vi "Process.vi"(0 "reference in":refnum<class "HPS-17000-PowerModule.lvclass">, 5 "error in":errorcluster) -> (14 "reference out":refnum<class "HPS-17000-PowerModule.lvclass">, 19 "error out":errorcluster)   [LabVIEW 2023, in "HPS-17000-PowerModule.lvlib" / "HPS-17000-PowerModule.lvclass"]
uses:
  HPS-17000-PowerModule.lvclass
  HPS-17000-PowerModule.lvclass/HPS-17000-PowerModule.ctl
  <vilib>/Utility/SystemLogging/NI_SystemLogging.lvlib
  <instrlib>/HPS-17000/Client Facing Datatypes/Setpoint Stream Status Data.ctl
  <instrlib>/HPS-17000/HPS-17000.lvclass
  <instrlib>/HPS-17000/Client Facing Datatypes/Network Sync Event Data.ctl
  <instrlib>/HPS-17000/Client Facing Datatypes/Faults Event Data.ctl
  <instrlib>/HPS-17000/Client Facing Datatypes/Heartbeat Event Data.ctl
  <instrlib>/HPS-17000/Client Facing Datatypes/Multi-Cycler Events.ctl
  SSH_class/SSH.lvclass
  private/Get XC Report.vi
  private/Search HPS Network.vi
  <vilib>/HPS-17000/nibatterycycler_grpc_Setpoint.ctl
  <vilib>/HPS-17000/NI_BC_client.lvlib
  <instrlib>/HPS-17000/Client Facing Datatypes/DeviceProperties.ctl
  builds/PowerModuleInterface/PowerModuleInterface.lvlibp/Classes/PowerModule_interface/Slew Rates.ctl
  builds/PowerModuleInterface/PowerModuleInterface.lvlibp/Classes/PowerModule_interface/PowerModuleInterface.lvclass
  <instrlib>/HPS-17000/Internal/Identify Multi.vi
  <instrlib>/HPS-17000/Internal/Get Status Multi.vi
  <instrlib>/HPS-17000/Internal/Start Measurement Stream Multi.vi
  <instrlib>/HPS-17000/Internal/Start Setpoint Stream Multi.vi
  <instrlib>/HPS-17000/Internal/Stream Setpoints Multi.vi
  <instrlib>/HPS-17000/Internal/Stop Setpoint Stream Multi.vi
  <instrlib>/HPS-17000/Internal/Stop Measurement Stream Multi.vi
panel:
  in  "Main Tab Control":T1(tab)
  in  "TSN NIC IP Address":string caption="TSN NIC IP ADDRESS"
  in  "Controller TSN IP":string caption="CONTROLLER TSN IP"
  in  "HPS17K Search":bool
  in  "Device Search":string(tree) caption="HPS17K SEARCH"
  in  "HPS17K IP Addresses":string[](tree) caption="HPS17K NETWORK"
  in  "Add HPS17K":bool
  in  "Remove HPS17K":bool
  in  "HPS Topology":enum16{"SINGLE", "MULTI"}(ring) caption="HPS17K TOPOLOGY"
  out "Self Test Log":i32(listbox) caption="SELF TEST LOG"
  in  "Run Self Test":bool
  out "Test Server Log":i32(listbox) caption="TEST SERVER LOG"
  in  "Run Test Server":bool
  in  "Voltage Reformation":bool caption="REFORMATION"
  in  "Get Device Properties":bool
  in  "Get XC Report":bool
  out "Event Log":i32(listbox)=-1 caption="EVENT LOG"
  in  "Clear Event Log":bool
  in  "Volta Monitor":bool
  out "device properties":T2
  out "GM ID":string
  out "Measurement Stream":bool caption="MEASUREMENT STREAM"
  out "Setpoint Stream":bool caption="SETPOINT STREAM"
  out "OK":bool
  out "Heartbeat Valid":bool caption="HEARTBEAT VALID"
  in  "FC Sys Inspect":bool
  out "Fault Description":string caption="FAULT DESCRIPTION"
  in  "Update Temperatures":bool
  out "Temperatures":i32(listbox) caption="TEMPERATURES"
  out "Thermal Limits":i32(listbox) caption="THERMAL LIMITS"
  out "Hardware Limits":i32(listbox) caption="HARDWARE LIMITS"
  out "Last Command":string
  out "error info":errorcluster
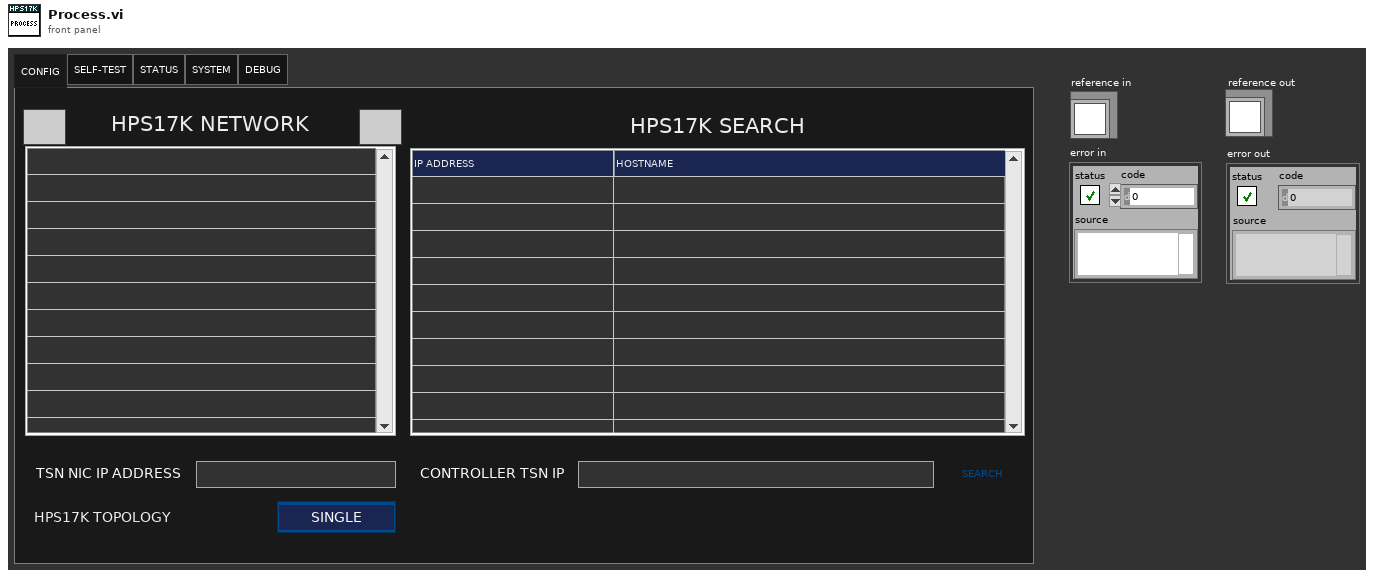
[diagram p1: front panel]
types:
  T1 = enum32{"CONFIG", "SELF-TEST", "STATUS", "SYSTEM", "DEBUG"}
  T2 = typedef "HPS-17000.lvclass/DeviceProperties.ctl" = cluster{"name":string, "model":string, "vendor":string, "serial_number":string}
  T3 = cluster{"Core":cluster{"Timeout":i32, "Events":cluster{"EventsToProcess":refnum<event-registration>, "UserEvents":refnum<event-registration>}, "EventFromProcess":refnum<user-event>, "ProcessSyncQueue":refnum<queue>, "QueueFromProcess":refnum<queue>, "Command":string, "Data":variant}, "Test Server":refnum<class "SSH.lvclass">, "Self Test":refnum<class "SSH.lvclass">, "Self Test Completed":refnum<user-event>, "Network Search Completed":refnum<user-event>, "Drag Data":cluster{"data name":string, "drag data":variant}[]}
  T4 = cluster{"data name":string, "drag data":variant}[]
  T5 = enum32{"Invalid", "Standard", "Closed", "Hidden", "Minimized", "Maximized"}
  T6 = enum8{"Enabled", "Disabled", "Disabled and Grayed Out"}
  T7 = typedef "NI_BC_client.lvlib/nibatterycycler_grpc_Setpoint.ctl" = cluster{"voltage":sgl, "current":sgl, "min_power":sgl, "max_power":sgl, "resistance":sgl}
  T8 = typedef "PowerModuleInterface.lvlibp/PowerModuleInterface.lvclass/Slew Rates.ctl" = cluster{"Current Decrease (A/sec)":dbl, "Current Increase (A/sec)":dbl, "Voltage Decrease (V/sec)":dbl, "Voltage Increase (V/sec)":dbl, "Resistance Decrease (Ohm/sec)":dbl, "Resistance Increase (Ohm/sec)":dbl}
  T9 = cluster{"EventsToProcess":refnum<event-registration>, "UserEvents":refnum<event-registration>}
  T10 = typedef "HPS-17000-PowerModule.lvlib/HPS-17000-PowerModule.lvclass/ObjectAttributes.ctl" = cluster{"JSON Config Path":path, "Configuration":T11, "GM ID":string, "HPS17000 Refs":refnum<class "HPS-17000.lvclass">[], "connected":bool, "reserved":bool, "events":T13, "nibatterycycler_grpc_Setpoint":T7, "last timestamp":i64, "mode":T14, "range":T15, "measurement array":T16[], "measurement stream":bool, "setpoint stream":bool}
  T11 = typedef "HPS-17000-PowerModule.lvlib/HPS-17000-PowerModule.lvclass/Configuration.ctl" = cluster{"TSN NIC IP Address":string, "HPS17000 IP Addresses":string[], "HPS Topology":enum16{"SINGLE", "MULTI"}, "Setpoint Stream Config":T12, "Measurement Array Size":i32, "Read Timeout (ms)":i32}
  T12 = typedef "Cycler.lvclass/Setpoint Stream Basic Config.ctl" = cluster{"local address":string, "receiver port":u16}
  T13 = typedef "HPS-17000.lvclass/Multi-Cycler Events.ctl" = cluster{"heartbeats events":refnum<user-event>[], "faults events":refnum<user-event>[], "network sync event":refnum<user-event>[], "setpoint status event":refnum<user-event>[]}
  T14 = typedef "HPS-17000-PowerModule.lvlib/HPS-17000-PowerModule.lvclass/Mode.ctl" = u16
  T15 = typedef "PowerModuleInterface.lvlibp/PowerModuleInterface.lvclass/Range.ctl" = cluster{"Current Max (A)":dbl, "Current Min (A)":dbl, "Voltage Max (V)":dbl, "Voltage Min (V)":dbl}
  T16 = typedef "PowerModuleInterface.lvlibp/PowerModuleInterface.lvclass/Measurements.ctl" = cluster{"measured voltage (V)":dbl, "measured current (A)":dbl, "setpoint voltage (V)":dbl, "setpoint current (A)":dbl, "timestamp":dbl}
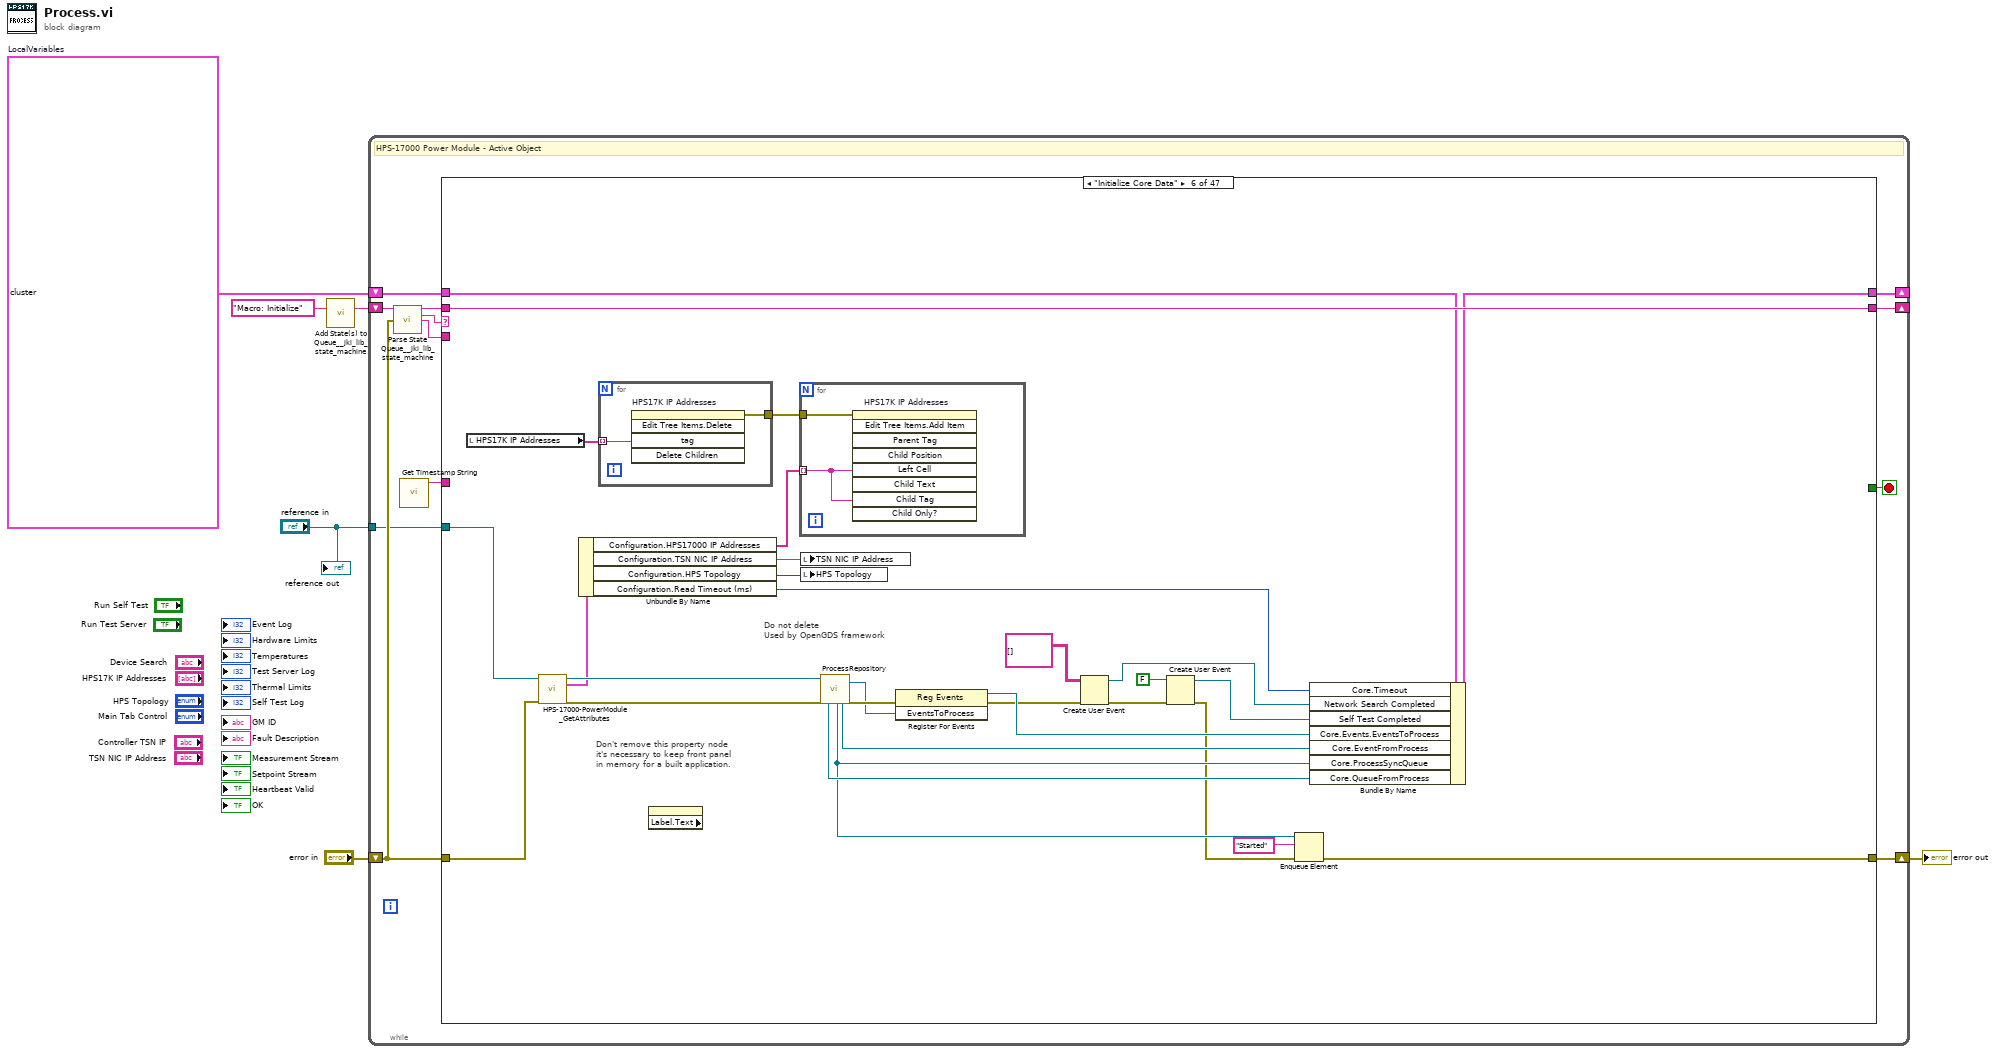
[diagram p0: block diagram]
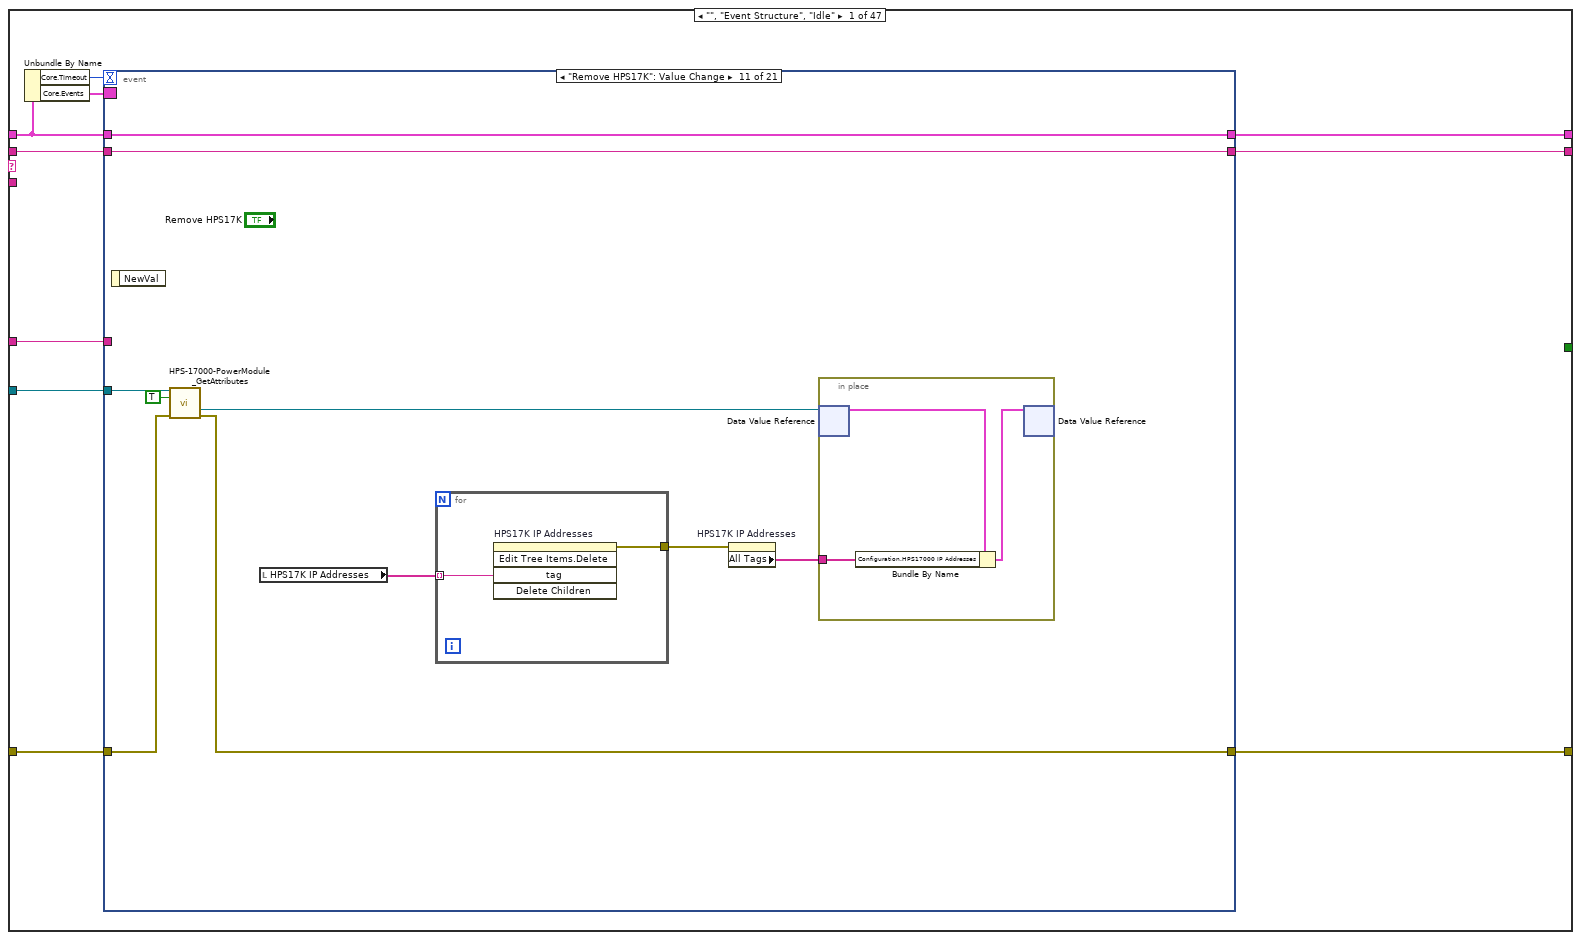
[diagram p2: hidden frame]
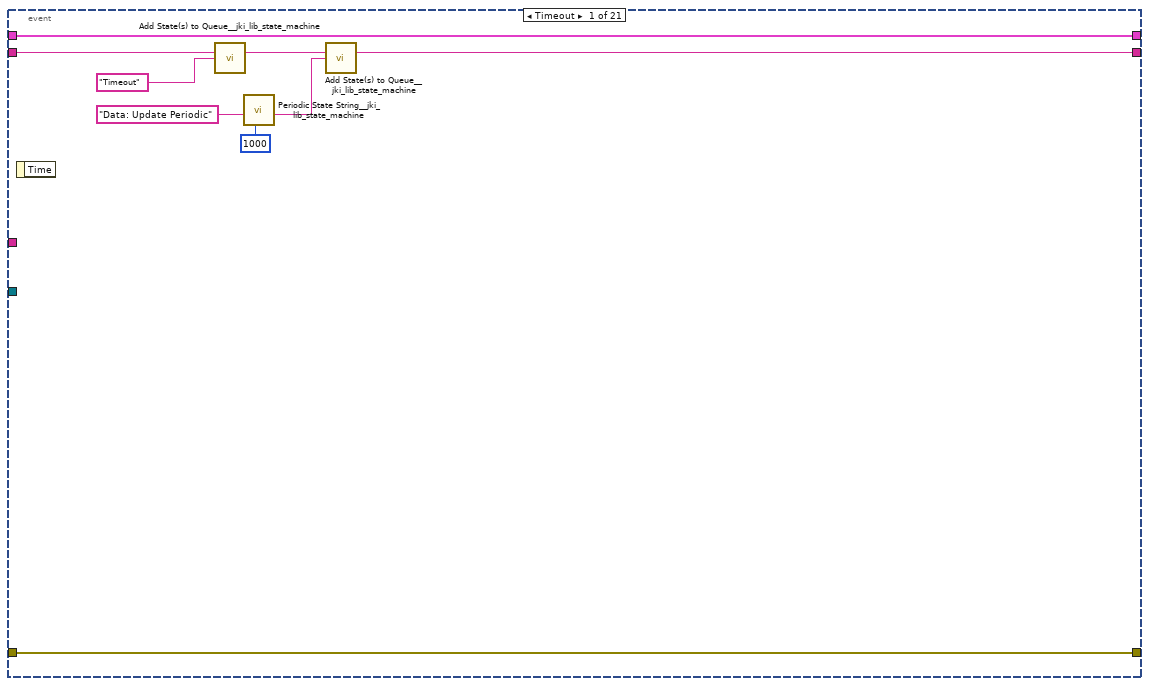
[diagram p3: hidden frame]
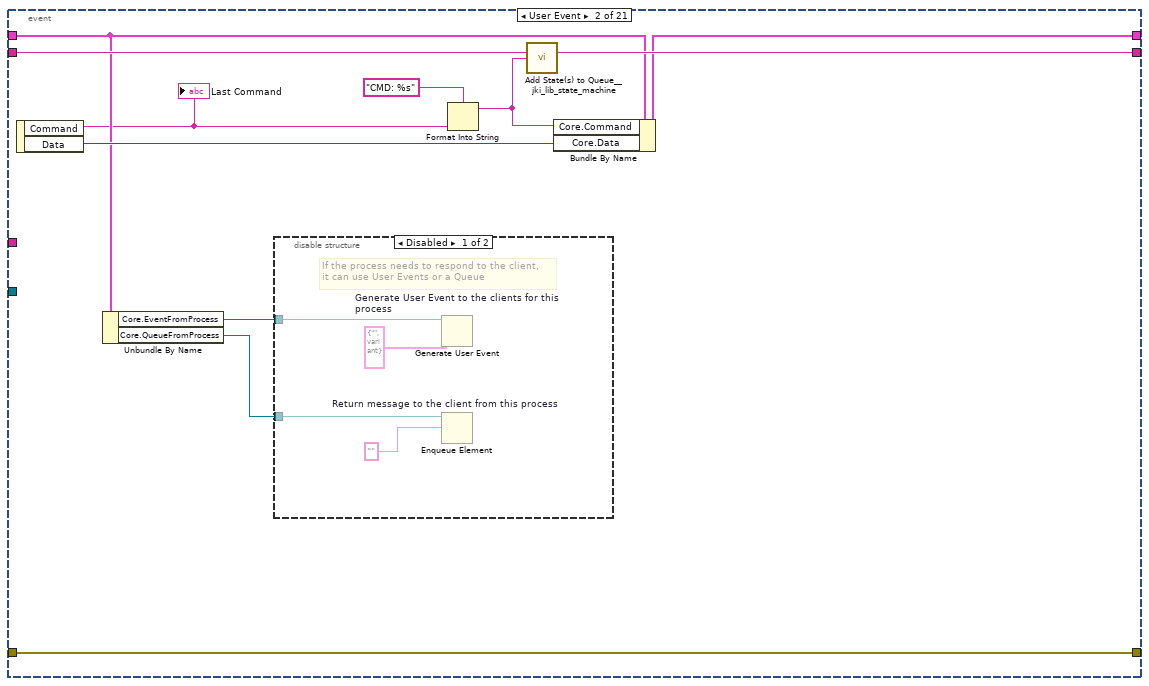
[diagram p4: hidden frame]
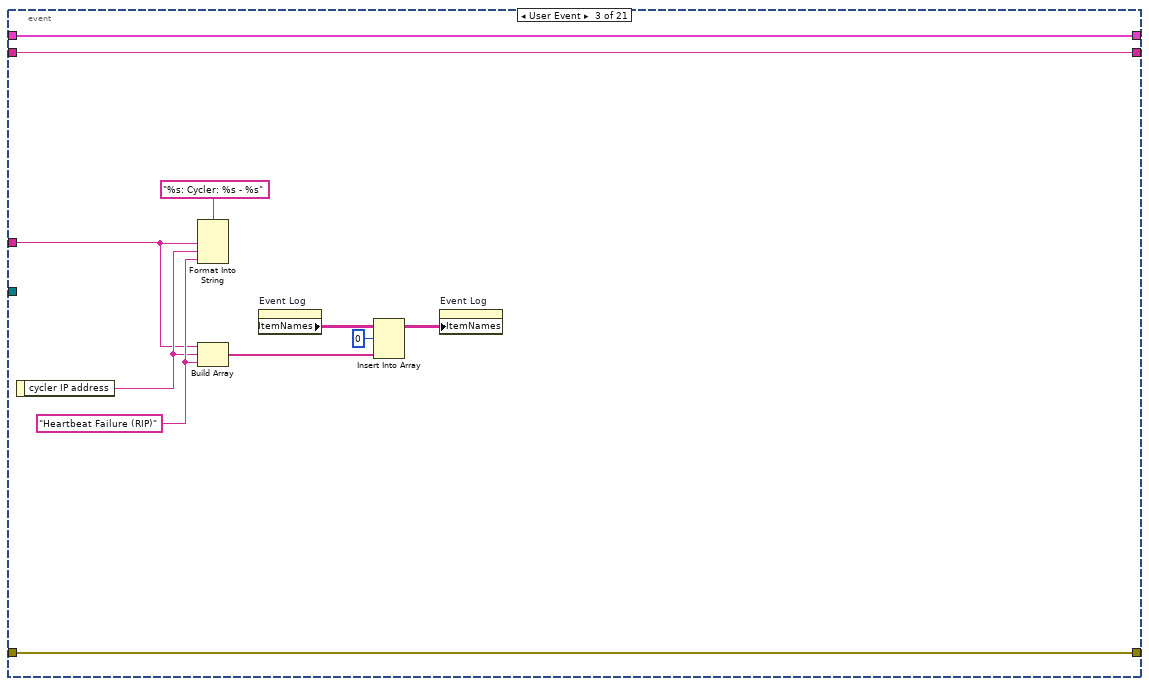
[diagram p6: hidden frame]
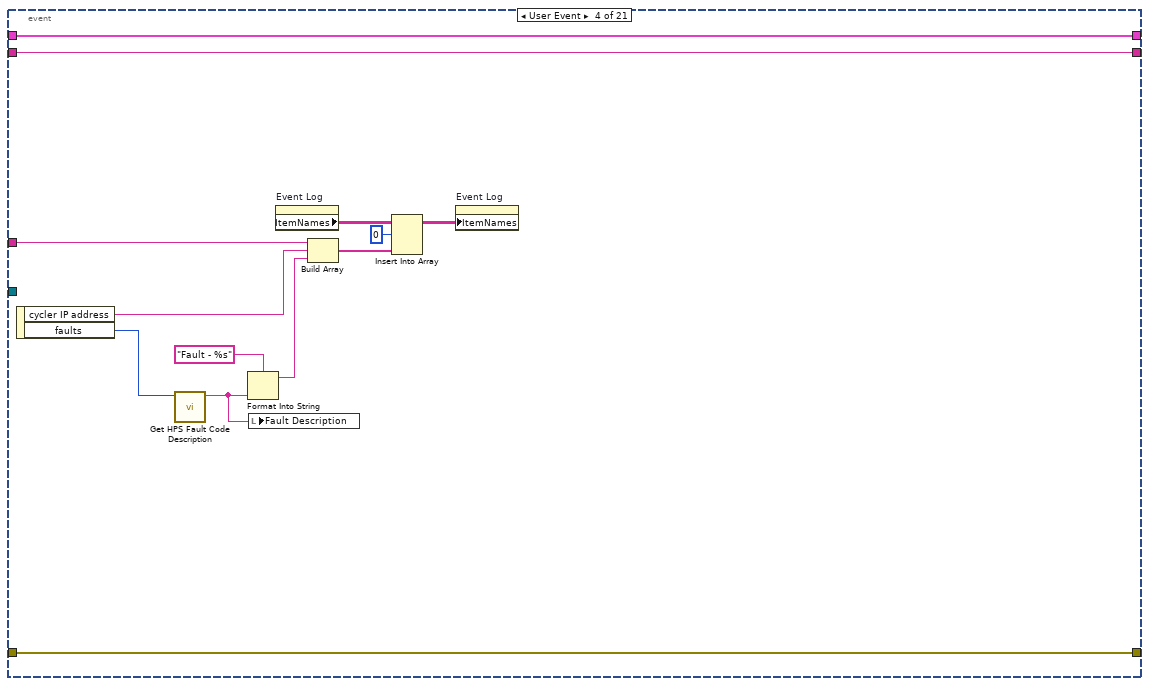
[diagram p7: hidden frame]
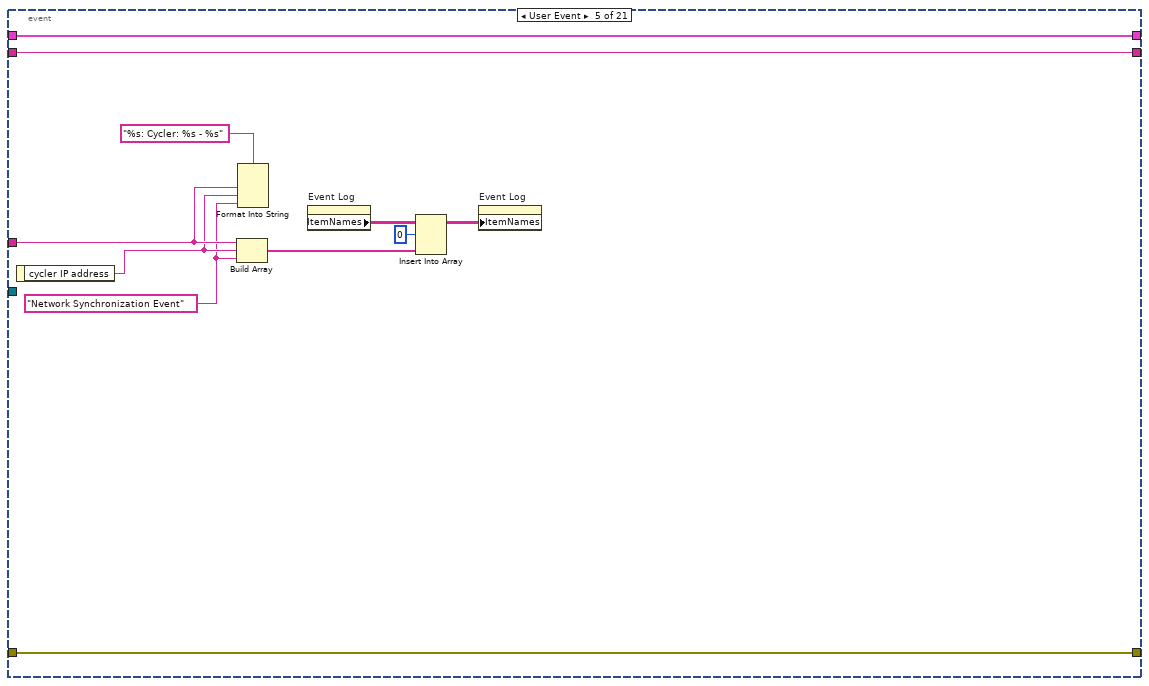
[diagram p8: hidden frame]
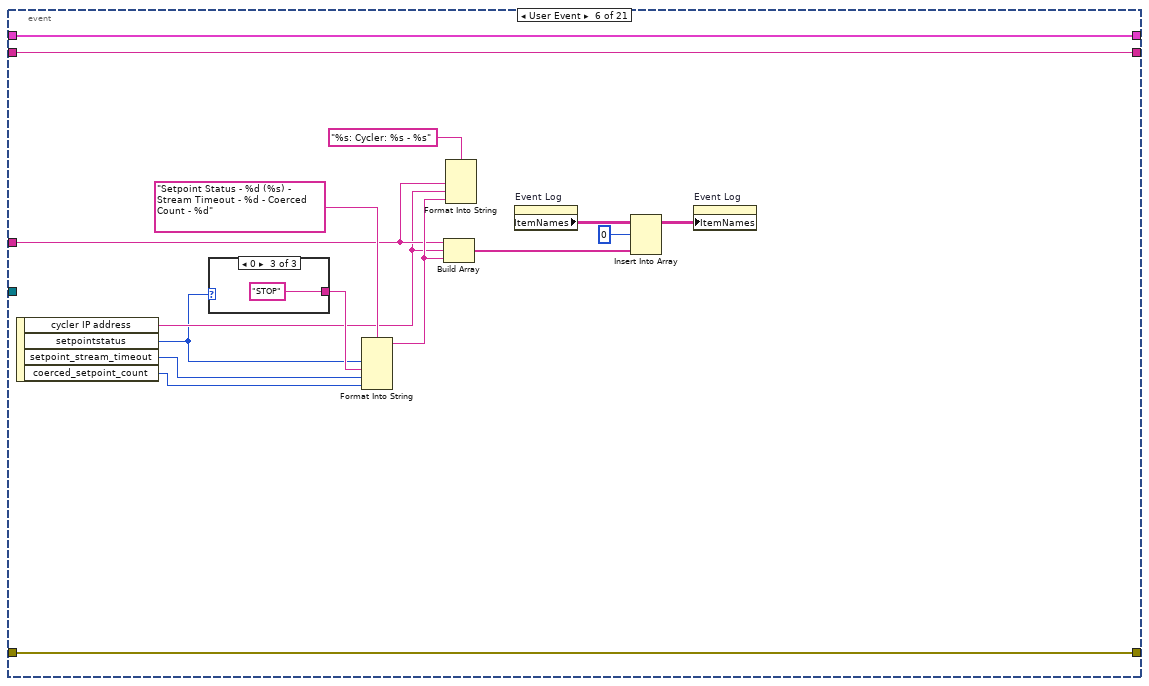
[diagram p9: hidden frame]
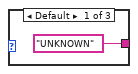
[diagram p10: hidden frame]
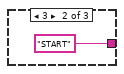
[diagram p11: hidden frame]
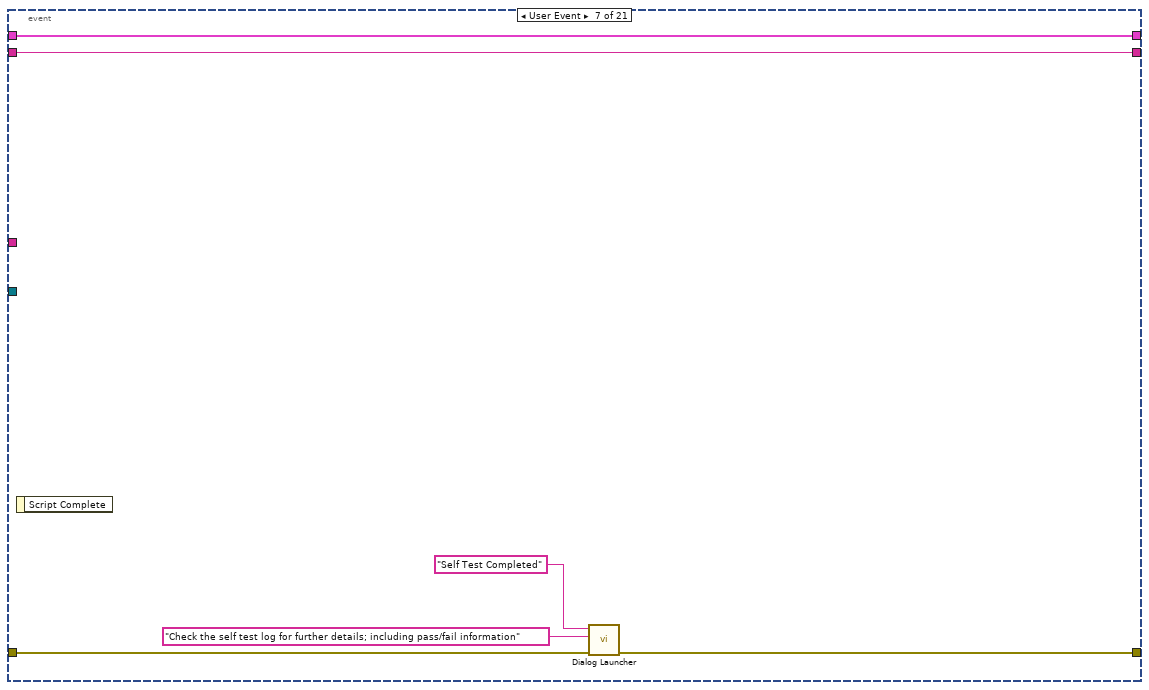
[diagram p12: hidden frame]
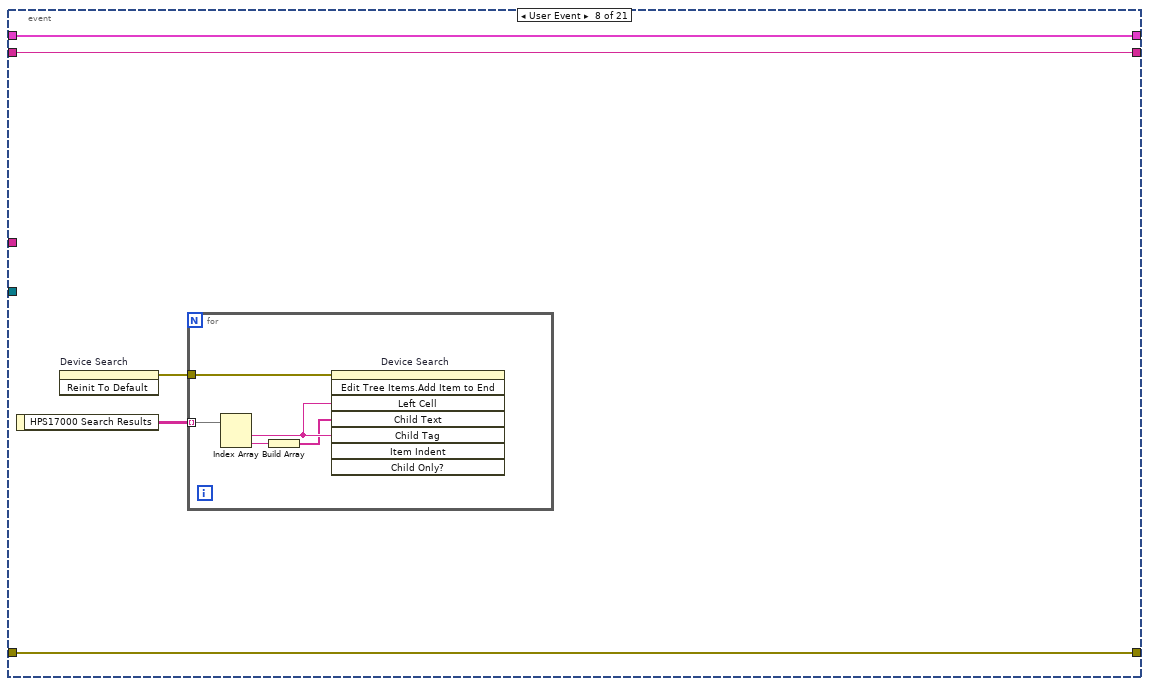
[diagram p13: hidden frame]
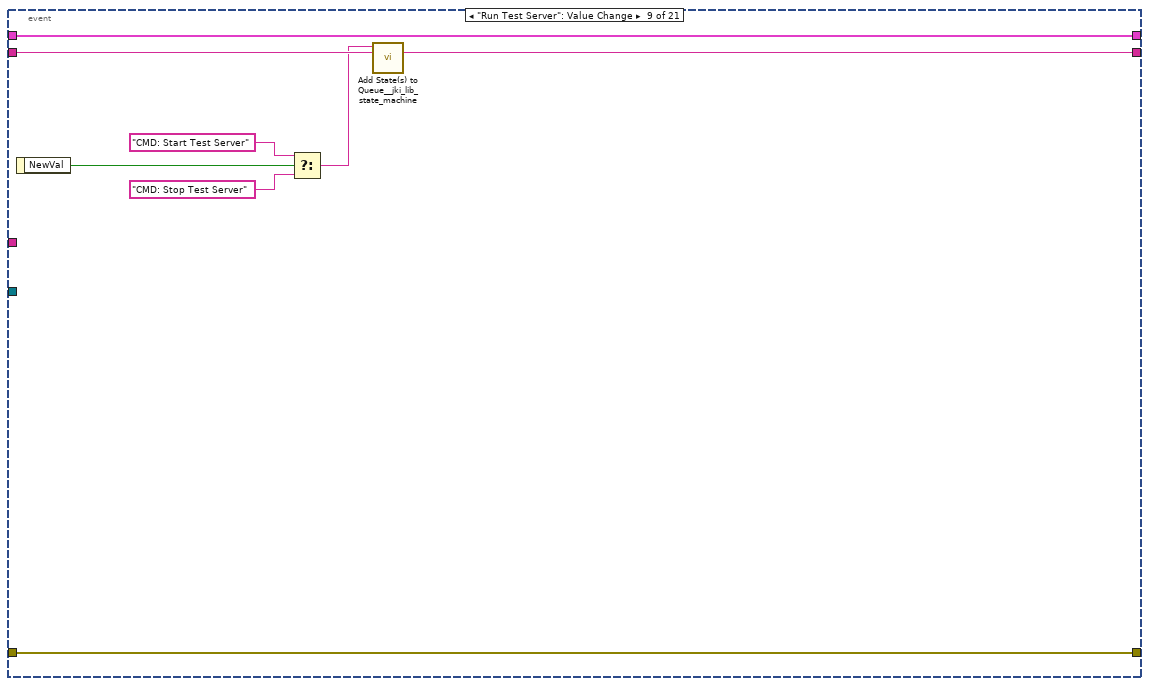
[diagram p14: hidden frame]
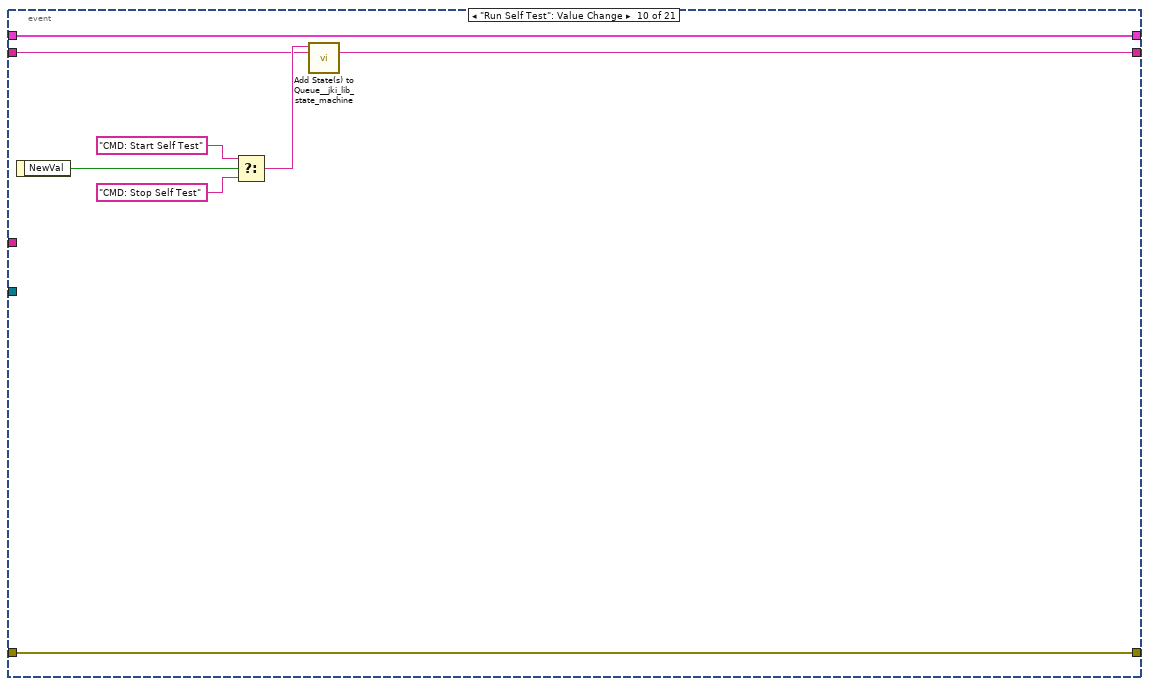
[diagram p15: hidden frame]
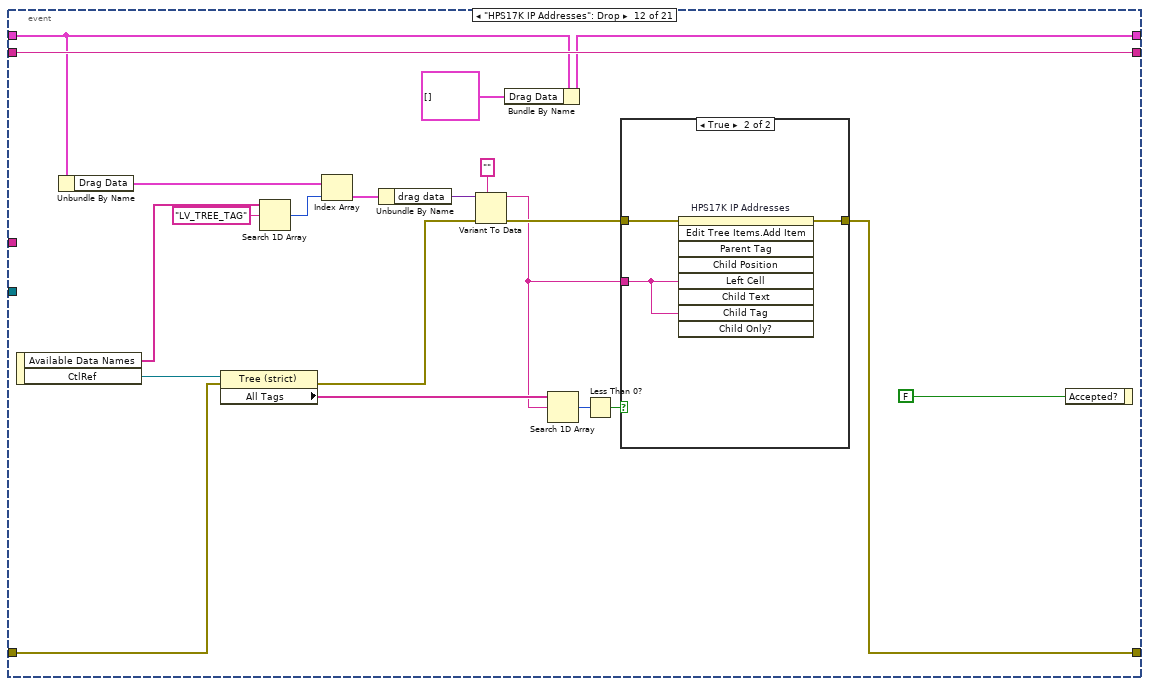
[diagram p16: hidden frame]
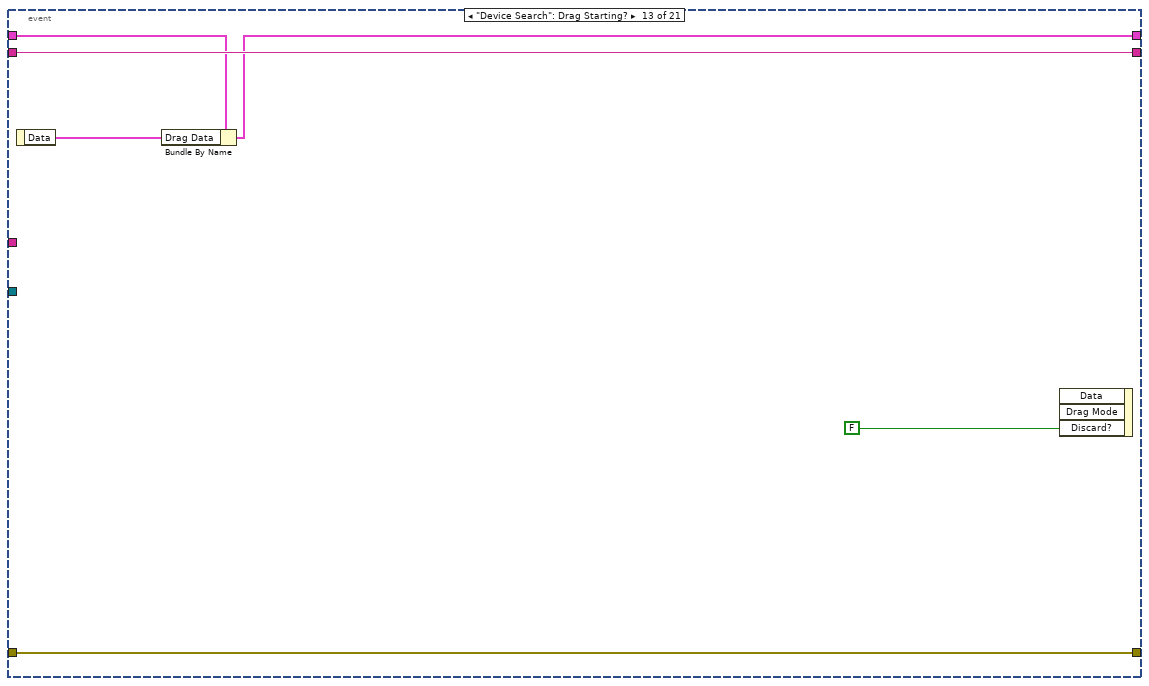
[diagram p18: hidden frame]
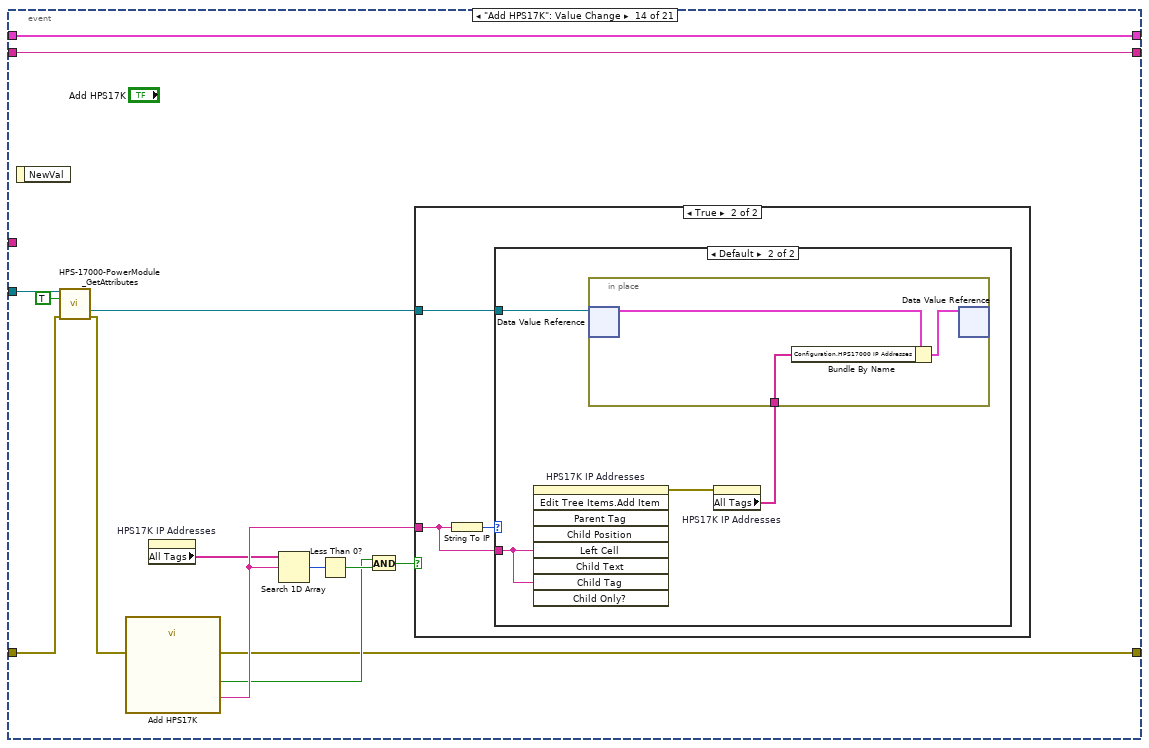
[diagram p19: hidden frame]
diagram:
  w6 = T3 {"Core"={"Timeout"=-1, "Events"={"EventsToProcess"=refnum, "UserEvents"=refnum}, "EventFromProcess"=refnum, "ProcessSyncQueue"=refnum, "QueueFromProcess"=refnum, "Command"="", "Data"=variant}, "Test Server"=refnum, "Self Test"=refnum, "Self Test Completed"=refnum, "Network Search Completed"=refnum, "Drag Data"=[]}  # LocalVariables
  n1 = call <vilib>:"Add State(s) to Queue__jki_lib_state_machine.vi"("State(s) in (\"\")"="Macro: Initialize" ("States Out")) -> ("States Out"=w2:string)  [unwired: 14 in]
  n2 = while {
    shift-right: [w17] -> w5
    shift-left: "error in" -> [w18]
    shift-right: [w10] -> _
    shift-left: w2 -> [w13]
    shift-right: [w16] -> _
    shift-left: w6 -> [w15]
    tunnel: "reference in" -> [w8]
    stop <- w9 stop-if-true
    # "HPS-17000 Power Module - Active Object"
    n3 = call <vilib>:"Parse State Queue__jki_lib_state_machine.vi"("State Queue"=w13, "Error In (no error)"=w18) -> ("Remaining States"=w12:string, "Current State"=w14:string, "Arguments"=w11:string)  [unwired: 11 in]
    n4 = call "Get Timestamp String.vi"() -> ("date/time string"=w7:string)  [unwired: 11 in]
    n5 = case shown="\"Initialize Core Data\"" w14 {
      selector: w14 -> [_ _ w291 _ _ _ _ _ _ _ _ _ _ _ _ _ _ _ _ _ _ _ _ _ _ _ _ _ _ _ _ _ _ _ _ _ _ _ _ _ _ _ _ _ _ _ _]
      tunnel: w18 -> [w24 w290 w293 w313 w382 w399 w418 w442 w455 w456 w486 _ w492 w506 w510 w514 w519 w524 w527 w534 w539 w554 w581 w604 w634 w661 w677 w701 w729 w745 w758 w766 w777 w795 w814 w822 w838 w841 w846 w851 w856 w861 w866 w871 w876 w881 w886]
      tunnel: [w22 w290 w292 w308 errorcluster {"status"=FALSE, "code"=0, "source"=""} ("error constant") w413 w425 w438 w455 w456 w486 w487 w491 w506 w510 w514 w519 w524 w527 w534 w546 w553 w580 w601 w631 w658 w674 w698 w725 w741 w757 w765 w776 w782 w817 w825 w838 w841 w846 w851 w856 w861 w866 w871 w876 w881 w886] -> w17
      tunnel: [w28 w289 w300 w302 w384 w411 w426 w444 w454 w458 w478 w488 w495 w505 w509 w513 w518 w523 w526 w533 w544 w548 w579 w607 w637 w664 w680 w704 w724 w740 w763 w771 w779 w794 w819 w823 w837 w840 w845 w850 w855 w860 w865 w870 w875 w880 w885] -> w16
      tunnel: w15 -> [w25 w289 w300 w302 w384 w410 w426 w444 w454 w458 w478 w488 w495 w505 w509 w513 w518 w523 w526 w533 w545 w549 w578 w607 w637 w664 w680 w704 w723 w739 w763 w771 w779 w794 w819 w823 w837 w840 w845 w850 w855 w860 w865 w870 w875 w880 w885]
      tunnel: w12 -> [w27 w288 w299 w301 w383 w412 w429 w445 w453 w459 w485 w490 w494 w504 w508 w512 w517 w522 _ w532 w547 w555 w582 w606 w636 w663 w679 w703 w730 w746 w762 w770 w778 w797 w820 w824 w836 w839 w844 w849 w854 w859 w864 w869 w874 w879 w884]
      tunnel: w11 -> [_ _ _ _ _ _ _ _ _ w457 _ _ w493 _ _ _ _ _ _ w529 _ _ _ _ _ _ _ _ _ _ _ _ _ _ _ _ _ _ _ _ _ _ _ _ _ _ _]
      tunnel: [w26 w288 w299 w301 w383 w412 w429 w445 w453 w459 w485 w490 w494 w504 w508 w512 w516 w521 "Macro: Exit" ("State(s) at Back (\"\")") w531 w547 w555 w582 w606 w636 w663 w679 w703 w730 w746 w762 w770 w778 w797 w820 w824 w836 w839 w842 w848 w853 w858 w863 w868 w873 w878 w883] -> w10
      tunnel: [_ _ _ _ _ _ TRUE _ _ _ _ _ _ _ _ _ _ _ _ _ _ _ _ _ _ _ _ _ _ _ _ _ _ _ _ _ _ _ _ _ _ _ _ _ _ _ _] -> w9
      tunnel: w8 -> [w19 _ _ w314 _ w402 _ w443 _ _ _ _ _ _ _ _ _ _ _ _ w540 _ _ w605 w635 w662 w678 w702 _ _ _ _ _ _ _ w827 _ _ _ _ _ _ _ _ _ _ _]
      tunnel: w7 -> [w20 _ _ _ _ _ _ _ _ _ _ _ _ _ _ _ _ _ _ _ _ _ _ _ _ _ _ _ _ _ _ _ _ _ _ _ _ _ _ _ _ _ _ _ _ _ _]
      frame "", "Event Structure", "Idle" {
        n6 = Unbundle By Name(w25) -> ("Core.Timeout"=w23:i32, "Core.Events"=w21:T9)
        n7 = event shown="[10] \"Remove HPS17K\": Value Change" {
          selector: w21 -> [_ _ _ _ _ _ _ _ _ _ _ _ _ _ _ _ _ _ _ _ _]
          dyn-events: _ -> [_ _ _ _ _ _ _ _ _ _ _ _ _ _ _ _ _ _ _ _ _]
          timeout: w23 -> [_ _ _ _ _ _ _ _ _ _ _ _ _ _ _ _ _ _ _ _ _]
          tunnel: w25 -> [w37 w41 w63 w76 w87 w103 w112 w117 w130 w138 w148 w161 w181 w198 w218 w228 w238 w245 w278 w282 w287]
          tunnel: [w37 w46 w63 w76 w87 w103 w112 w117 w130 w138 w148 w160 w180 w198 w218 w228 w238 w245 w278 w282 w287] -> w28
          tunnel: [w29 w48 w62 w75 w86 w102 w111 w116 w127 w131 w147 w174 w184 w197 w217 w227 w237 w247 w274 w281 w283] -> w26
          tunnel: w27 -> [w36 w47 w62 w75 w86 w102 w111 w116 w128 w132 w147 w174 w184 w197 w217 w227 w237 w247 w276 w281 w285]
          tunnel: [w34 w42 w61 w74 w85 w101 w107 w115 w129 w137 w143 w154 w183 w191 w215 w226 w235 w246 w277 w280 w286] -> w22
          tunnel: w24 -> [w34 w42 w61 w74 w85 w101 w110 w115 w129 w137 w144 w167 w183 w188 w216 w224 w236 w241 w277 w280 w286]
          tunnel: w20 -> [_ _ w53 w66 w80 w94 _ _ _ _ _ _ _ _ _ _ _ _ _ _ _]
          tunnel: w19 -> [_ _ _ _ _ _ _ _ _ _ w146 _ _ w189 _ w225 _ w242 _ _ _]
          event Timeout {
            n8 = event-data() -> ()  [unwired: 1 in, 1 out]
            n9 = call <vilib>:"Add State(s) to Queue__jki_lib_state_machine.vi"("State(s) in (\"\")"=w36, "State(s) at Back (\"\")"="Timeout" ("State(s) at Back (\"\")")) -> ("States Out"=w32:string)  [unwired: 13 in]
            n10 = call <vilib>:"Periodic State String__jki_lib_state_machine.vi"("Period (ms)"=u32 1000, "State"="Data: Update Periodic") -> ("State Out"=w31:string)  [unwired: 9 in]
            n11 = call <vilib>:"Add State(s) to Queue__jki_lib_state_machine.vi"("State(s) in (\"\")"=w32, "State(s) at Back (\"\")"=w31) -> ("States Out"=w29:string)  [unwired: 13 in]
          }
          event User Event {
            n12 = event-data() -> ("Command"=w39:string, "Data"=w45:variant)  [unwired: 1 in]
            "Last Command" <- w39
            n13 = Unbundle By Name(w41) -> ("Core.EventFromProcess"=w44:refnum<user-event>, "Core.QueueFromProcess"=w43:refnum<queue>)
            n14 = disable-structure shown="Disabled" {
              disable-tunnel: w44 -> [w52 _]
              disable-tunnel: w43 -> [w51 _]
              frame Disabled {
                # "If the process needs to respond to the client,\nit can use User Events or a Queue"
                n15 = Generate User Event "Generate User Event to the clients for this process"(user event=w52, event data cluster=cluster{"Command":string, "Data":variant} {"Command"="", "Data"=variant} ("event data")) -> ()  [unwired: 2 in, 2 out]
                n16 = Enqueue Element "Return message to the client from this process"(queue=w51, element="") -> ()  [unwired: 2 in, 3 out]
              }
              frame Enabled {
              }
            }
            n17 = Format Into String(format string="CMD: %s", w39) -> (resulting string=w38:string)  [unwired: 2 in, 1 out]
            n18 = call <vilib>:"Add State(s) to Queue__jki_lib_state_machine.vi"("State(s) in (\"\")"=w47, "State(s) at Back (\"\")"=w38) -> ("States Out"=w48:string)  [unwired: 13 in]
            n19 = Bundle By Name(cluster=w41, "Core.Command"=w38, "Core.Data"=w45) -> (w46:T3)
          }
          event User Event {
            w56 = "Heartbeat Failure (RIP)" ("format string")
            n20 = event-data() -> ("cycler IP address"=w55:string)  [unwired: 1 in]
            n21 = Format Into String(format string="%s: Cycler: %s - %s", w53, w55, w56) -> ()  [unwired: 2 in, 2 out]
            n22 = Build Array(w53, w55, w56) -> (w59:string[])
            n23 = property on="Event Log" class="MCListbox (strict)"() -> ("ItemNames"=w60:string[][])  [unwired: 2 in, 2 out]
            n24 = Insert Into Array(array=w60, index (row)=0, new element=w59) -> (w54:string[][])  [unwired: 1 in]
            n25 = property on="Event Log" class="MCListbox (strict)"("ItemNames"=w54) -> ()  [unwired: 2 in, 2 out]
          }
          event User Event {
            n26 = event-data() -> ("cycler IP address"=w67:string, "faults"=w68:u64)  [unwired: 1 in]
            n27 = call "Get HPS Fault Code Description.vi"("fault code"=w68) -> ("fault description"=w69:string)  [unwired: 10 in]
            n28 = Format Into String(format string="Fault - %s", w69) -> (resulting string=w72:string)  [unwired: 2 in, 1 out]
            n29 = local write "Fault Description"(w69) -> ()
            n30 = property on="Event Log" class="MCListbox (strict)"() -> ("ItemNames"=w65:string[][])  [unwired: 2 in, 2 out]
            n31 = Build Array(w66, w67, w72) -> (w70:string[])
            n32 = Insert Into Array(array=w65, index (row)=0, new element=w70) -> (w64:string[][])  [unwired: 1 in]
            n33 = property on="Event Log" class="MCListbox (strict)"("ItemNames"=w64) -> ()  [unwired: 2 in, 2 out]
          }
          event User Event {
            w78 = "Network Synchronization Event" ("format string")
            n34 = event-data() -> ("cycler IP address"=w79:string)  [unwired: 1 in]
            n35 = Build Array(w80, w79, w78) -> (w77:string[])
            n36 = Format Into String(format string="%s: Cycler: %s - %s", w80, w79, w78) -> ()  [unwired: 2 in, 2 out]
            n37 = property on="Event Log" class="MCListbox (strict)"() -> ("ItemNames"=w84:string[][])  [unwired: 2 in, 2 out]
            n38 = Insert Into Array(array=w84, index (row)=0, new element=w77) -> (w83:string[][])  [unwired: 1 in]
            n39 = property on="Event Log" class="MCListbox (strict)"("ItemNames"=w83) -> ()  [unwired: 2 in, 2 out]
          }
          event User Event {
            n40 = event-data() -> ("cycler IP address"=w93:string, "setpointstatus"=w92:i32, "setpoint_stream_timeout"=w91:u32, "coerced_setpoint_count"=w90:u32)  [unwired: 1 in]
            n41 = case shown="0" w92 {
              tunnel: ["UNKNOWN" ("input 2") "START" ("input 2") "STOP" ("input 2")] -> w95
              frame Default {
              }
              frame 3 {
              }
              frame 0 {
              }
            }
            n42 = Format Into String(format string="Setpoint Status - %d (%s) - Stream Timeout - %d - Coerced Count - %d", w92, w95, w91, w90) -> (resulting string=w96:string)  [unwired: 2 in, 1 out]
            n43 = Build Array(w94, w93, w96) -> (w100:string[])
            n44 = Format Into String(format string="%s: Cycler: %s - %s", w94, w93, w96) -> ()  [unwired: 2 in, 2 out]
            n45 = property on="Event Log" class="MCListbox (strict)"() -> ("ItemNames"=w89:string[][])  [unwired: 2 in, 2 out]
            n46 = Insert Into Array(array=w89, index (row)=0, new element=w100) -> (w88:string[][])  [unwired: 1 in]
            n47 = property on="Event Log" class="MCListbox (strict)"("ItemNames"=w88) -> ()  [unwired: 2 in, 2 out]
          }
          event User Event {
            n48 = event-data() -> ()  [unwired: 1 in, 1 out]
            n49 = call "Dialog Launcher.vi"("error in (no error)"=w110, "Message"="Check the self test log for further details; including pass/fail information", "Title"="Self Test Completed") -> ("error out"=w107:errorcluster)  [unwired: 8 in]
          }
          event User Event {
            n50 = event-data() -> ("HPS17000 Search Results"=w113:string[][])  [unwired: 1 in]
            n51 = invoke on="Device Search" class="Tree (strict)" method="Reinit To Default"() -> (error out=w114:errorcluster)  [unwired: 3 in, 2 out]
            n52 = for {
              tunnel: w114 -> [w122]
              tunnel: w113 -> [w121] mode=indexing
              n53 = Index Array(array=w121) -> (element #1=w120:string, element #2=w119:string)  [unwired: 2 in]
              n54 = Build Array(w119) -> (w118:string[])
              n55 = invoke on="Device Search" class="Tree (strict)" method="Edit Tree Items.Add Item to End"(error in=w122, "Left Cell"=w120, "Child Text"=w118, "Child Tag"=w120) -> ()  [unwired: 4 in, 8 out]
            }
          }
          event "Run Test Server": Value Change {
            n56 = event-data() -> ("NewVal"=w125:bool)  [unwired: 1 in]
            n57 = Select(t="CMD: Start Test Server" ("State(s) in Front (\"\")"), s=w125, f="CMD: Stop Test Server" ("State(s) in Front (\"\")")) -> (s? t:f=w123:string)
            n58 = call <vilib>:"Add State(s) to Queue__jki_lib_state_machine.vi"("State(s) in Front (\"\")"=w123, "State(s) in (\"\")"=w128) -> ("States Out"=w127:string)  [unwired: 13 in]
          }
          event "Run Self Test": Value Change {
            n59 = event-data() -> ("NewVal"=w134:bool)  [unwired: 1 in]
            n60 = Select(t="CMD: Start Self Test" ("State(s) in Front (\"\")"), s=w134, f="CMD: Stop Self Test" ("State(s) in Front (\"\")")) -> (s? t:f=w133:string)
            n61 = call <vilib>:"Add State(s) to Queue__jki_lib_state_machine.vi"("State(s) in Front (\"\")"=w133, "State(s) in (\"\")"=w132) -> ("States Out"=w131:string)  [unwired: 13 in]
          }
          event "Remove HPS17K": Value Change {
            n62 = event-data() -> ()  [unwired: 1 in, 1 out]
            n63 = call "HPS-17000-PowerModule_GetAttributes.vi"("reference in"=w146, "OnlyGetDvrReference(False)"=TRUE, "Error In"=w144) -> ("DataRef"=w140:refnum<data-value>, "Error Out"=w143:errorcluster)  [unwired: 9 in, 2 out]
            n64 = local read "HPS17K IP Addresses"() -> (w142:string[])
            n65 = for {
              tunnel: w142 -> [w153] mode=indexing
              tunnel: [w152] -> w141
              n66 = invoke on="HPS17K IP Addresses" class="Tree (strict)" method="Edit Tree Items.Delete"("tag"=w153) -> (error out=w152:errorcluster)  [unwired: 4 in, 4 out]
            }
            n67 = property on="HPS17K IP Addresses" class="Tree (strict)"(error in=w141) -> ("All Tags"=w139:string[])  [unwired: 1 in, 2 out]
            n68 = in-place {
              in-place-border: w139 -> [w149]
              n69 = in-place-dvr #1(w140) -> (w151:T10)  [unwired: 1 out]
              n70 = Bundle By Name(cluster=w151, "Configuration.HPS17000 IP Addresses"=w149) -> (w150:T10)
              n71 = in-place-dvr #1(w150) -> ()  [unwired: 2 out]
            }
          }
          event "HPS17K IP Addresses": Drop {
            n72 = event-data() -> ("Available Data Names"=w173:string[], "CtlRef"=w168:refnum<vi>)  [unwired: 1 in]
            n73 = Unbundle By Name(w161) -> ("Drag Data"=w171:T4)
            n74 = property class="Tree (strict)"(reference=w168, error in=w167) -> (error out=w166:errorcluster, "All Tags"=w163:string[])  [unwired: 1 out]
            n75 = Search 1D Array(1D array=w173, element="LV_TREE_TAG") -> (index of element=w170:i32)  [unwired: 1 in]
            n76 = Index Array(array=w171, index=w170) -> (element=w169:cluster{"data name":string, "drag data":variant})
            n77 = Unbundle By Name(w169) -> ("drag data"=w165:variant)
            n78 = Variant To Data(error in=w166, type="", Variant=w165) -> (data=w155:string, error out=w158:errorcluster)
            n79 = Bundle By Name(cluster=w161, "Drag Data"=T4 []) -> (w160:T3)
            n80 = Search 1D Array(1D array=w163, element=w155) -> (index of element=w157:i32)  [unwired: 1 in]
            n81 = Less Than 0?(x=w157) -> (x < 0?=w156:bool)
            n82 = case shown="True" w156 {
              tunnel: w158 -> [w175 w178]
              tunnel: w155 -> [_ w177]
              tunnel: [w175 w176] -> w154
              frame False {
              }
              frame True {
                n83 = invoke on="HPS17K IP Addresses" class="Tree (strict)" method="Edit Tree Items.Add Item"(error in=w178, "Left Cell"=w177, "Child Tag"=w177) -> (error out=w176:errorcluster)  [unwired: 6 in, 8 out]
              }
            }
            n84 = event-data("Accepted?"=FALSE) -> ()  [unwired: 1 in, 1 out]
          }
          event "Device Search": Drag Starting? {
            n85 = event-data() -> ("Data"=w179:T4)  [unwired: 1 in]
            n86 = Bundle By Name(cluster=w181, "Drag Data"=w179) -> (w180:T3)
            n87 = event-data("Discard?"=FALSE) -> ()  [unwired: 3 in, 1 out]
          }
          event "Add HPS17K": Value Change {
            n88 = event-data() -> ()  [unwired: 1 in, 1 out]
            n89 = call "HPS-17000-PowerModule_GetAttributes.vi"("reference in"=w189, "OnlyGetDvrReference(False)"=TRUE, "Error In"=w188) -> ("DataRef"=w185:refnum<data-value>, "Error Out"=w187:errorcluster)  [unwired: 9 in, 2 out]
            n90 = call "Add HPS17K"("error in (no error)"=w187) -> ("IP Address"=w196:string, "Add"=w193:bool, "error out"=w191:errorcluster)  [unwired: 16 in]
            n91 = property on="HPS17K IP Addresses" class="Tree (strict)"() -> ("All Tags"=w190:string[])  [unwired: 2 in, 2 out]
            n92 = Search 1D Array(1D array=w190, element=w196) -> (index of element=w195:i32)  [unwired: 1 in]
            n93 = Less Than 0?(x=w195) -> (x < 0?=w194:bool)
            n94 = And(x=w193, y=w194) -> (x .and. y?=w192:bool)
            n95 = case shown="True" w192 {
              tunnel: w196 -> [_ w200]
              tunnel: w185 -> [_ w199]
              frame False {
              }
              frame True {
                n96 = String To IP(1:w200) -> (0:w201:u32)
                n97 = case shown="Default" w201 {
                  tunnel: w200 -> [_ w205]
                  tunnel: w199 -> [_ w204]
                  frame 0, 181174352 {
                    # "0 = invalid\n\n181174352 = empty (localhost?)"
                  }
                  frame Default {
                    n98 = invoke on="HPS17K IP Addresses" class="Tree (strict)" method="Edit Tree Items.Add Item"("Left Cell"=w205, "Child Tag"=w205) -> (error out=w203:errorcluster)  [unwired: 7 in, 8 out]
                    n99 = property on="HPS17K IP Addresses" class="Tree (strict)"(error in=w203) -> ("All Tags"=w202:string[])  [unwired: 1 in, 2 out]
                    n100 = in-place {
                      in-place-border: w202 -> [w206]
                      n101 = in-place-dvr #2(w204) -> (w208:T10)  [unwired: 1 out]
                      n102 = Bundle By Name(cluster=w208, "Configuration.HPS17000 IP Addresses"=w206) -> (w207:T10)
                      n103 = in-place-dvr #2(w207) -> ()  [unwired: 2 out]
                    }
                  }
                }
              }
            }
          }
          event "Volta Monitor": Value Change {
            n104 = event-data() -> ()  [unwired: 1 in, 1 out]
            n105 = property on="HPS17K IP Addresses" class="Tree (strict)"() -> ("All Tags"=w209:string[])  [unwired: 2 in, 2 out]
            n106 = Index Array(array=w209) -> (element=w210:string)  [unwired: 1 in]
            n107 = Format Into String(format string="plink -l admin %s -batch -t \"/usr/local/natinst/bin/volta_monitor\"", w210) -> (resulting string=w213:string)  [unwired: 2 in, 1 out]
            n108 = call <vilib>:"System Exec.vi"("run minimized? (F)"=FALSE, "wait until completion? (T)"=FALSE, "error in (no error)"=w216, "command line"=w213) -> ("error out"=w215:errorcluster)  [unwired: 4 in, 3 out]
          }
          event "Get Device Properties": Value Change {
            n109 = event-data() -> ()  [unwired: 1 in, 1 out]
            n110 = call "HPS-17000-PowerModule_GetAttributes.vi"("reference in"=w225, "Error In"=w224) -> ("Data"=w222:T10, "Error Out"=w223:errorcluster)  [unwired: 10 in, 2 out]
            n111 = Unbundle By Name(w222) -> ("HPS17000 Refs"=w221:refnum<class "HPS-17000.lvclass">[])
            n112 = call-poly <instrlib>:"Identify.vi"("error in"=w223, "cycler refs in"=w221) -> ("error out"=w226:errorcluster, "device properties"=w220:T2[])  [unwired: 7 in, 1 out]
            n113 = Index Array(array=w220) -> (element=→"device properties":T2)  [unwired: 1 in]
          }
          event "FC Sys Inspect": Value Change {
            n114 = event-data() -> ()  [unwired: 1 in, 1 out]
            n115 = property on="HPS17K IP Addresses" class="Tree (strict)"() -> ("All Tags"=w229:string[])  [unwired: 2 in, 2 out]
            n116 = Index Array(array=w229) -> (element=w230:string)  [unwired: 1 in]
            n117 = Format Into String(format string="plink -l admin %s -batch -t \"/usr/local/natinst/bin/fc_sys_inspect\"", w230) -> (resulting string=w234:string)  [unwired: 2 in, 1 out]
            n118 = call <vilib>:"System Exec.vi"("run minimized? (F)"=FALSE, "wait until completion? (T)"=FALSE, "error in (no error)"=w236, "command line"=w234) -> ("error out"=w235:errorcluster)  [unwired: 4 in, 3 out]
          }
          event "Get XC Report": Value Change {
            n119 = event-data() -> ()  [unwired: 1 in, 1 out]
            n120 = call "HPS-17000-PowerModule_GetAttributes.vi"("reference in"=w242, "Error In"=w241) -> ("Data"=w239:T10, "Error Out"=w240:errorcluster)  [unwired: 10 in, 2 out]
            n121 = Unbundle By Name(w239) -> ("HPS17000 Refs"=w244:refnum<class "HPS-17000.lvclass">[], "connected"=w243:bool)
            n122 = case shown="True" w243 {
              tunnel: w240 -> [w248 w258]
              tunnel: [w248 w259] -> w246
              tunnel: w244 -> [_ w249]
              frame False {
              }
              frame True {
                n123 = call "File Dialog2"("prompt"="Select a file path for the diagnostic report", "default name"="xc_report.zip", "error in"=w258, "pattern (all files)"="*.zip", "pattern label"="Compressed XC Report") -> ("selected path"=w250:path, "cancelled"=w257:bool, "error out"=w256:errorcluster)  [unwired: 7 in, 1 out]
                n124 = Or(x=w257, y=w256) -> (x .or. y?=w255:bool)
                n125 = case shown="False" w255 {
                  tunnel: [w263 w273] -> w259
                  tunnel: w256 -> [w271 w273]
                  tunnel: w250 -> [w264 _]
                  tunnel: w249 -> [w261 _]
                  frame False {
                    w262 = 60000  # timeout in ms (60000)
                    w267 = 128  # call & forget
                    n126 = vi-ref "HPS-17000-PowerModule.lvlib:HPS-17000-PowerModule.lvclass:Get XC Report.vi"() -> (w272:refnum<vi>)
                    n127 = property class="VI Interface Type 0"(reference=w272, error in=w271) -> (reference out=w269:refnum<vi>, error out=w270:errorcluster, "Path"=w268:path)
                    n128 = Index Array(array=w261) -> (element=w260:refnum<class "HPS-17000.lvclass">)  [unwired: 1 in]
                    n129 = Open VI Reference(type specifier VI Refnum (for type only)=w269, vi path=w268, options=w267, error in (no error)=w270) -> (vi reference=w266:refnum<vi>, error out=w265:errorcluster)  [unwired: 2 in]
                    n130 = call-by-ref "Start Asynchronous Call"(reference=w266, error in=w265, "timeout in ms (60000)"=w262, "selected path"=w264, "HPS-17000 in"=w260) -> (error out=w263:errorcluster)  [unwired: 7 in, 3 out]
                  }
                  frame True {
                  }
                }
              }
            }
          }
          event "Update Temperatures": Value Change {
            n131 = event-data() -> ()  [unwired: 1 in, 1 out]
            n132 = call <vilib>:"Add State(s) to Queue__jki_lib_state_machine.vi"("State(s) in Front (\"\")"="CMD: Read Temperatures" ("States Out"), "State(s) in (\"\")"=w276) -> ("States Out"=w274:string)  [unwired: 13 in]
          }
          event "Clear Event Log": Value Change {
            n133 = event-data() -> ()  [unwired: 1 in, 1 out]
            n134 = property on="Event Log" class="MCListbox (strict)"("ItemNames"=string[][] [] ("Item Names")) -> ()  [unwired: 2 in, 2 out]
          }
          event "HPS17K Search": Value Change {
            n135 = event-data() -> ()  [unwired: 1 in, 1 out]
            n136 = call <vilib>:"Add State(s) to Queue__jki_lib_state_machine.vi"("State(s) in Front (\"\")"="CMD: Search HPS Network" ("States Out"), "State(s) in (\"\")"=w285) -> ("States Out"=w283:string)  [unwired: 13 in]
          }
        }
      }
      frame "---------- Core ----------" {
      }
      frame Default {
        w297 = 42 items=["No error", "Argument error", "Memory is full", "Out of zone", "End of file", "File already open", "Generic file I/O error", "File not found", "File permission error", "Disk is full", "Duplicate path", "Too many files open", "System feature not enabled", "Resource file not found", "Cannot add resource", "Resource not found", "Image not found", "Image memory error", "Pen does not exist", "Config type invalid", "Config token not found", "Config parse error", "Config memory error", "Bad external code format", "Bad external code offset", "External code not present", "Null window", "Destroy window error", "Null menu", "Print aborted", "Bad print record", "Print driver error", "Windows error during printing", "Memory error during printing", "Print dialog error", "Generic print error", "Invalid device refnum", "Device not found", "Device parameter error", "Device unit error", "Cannot open device", "Device call aborted", "Generic error", "Cancelled by user", "Object ID too low", "Object ID too high", "Object not in heap", "Unknown heap", "Unknown object (invalid DefProc)", "Unknown object (DefProc not in table)", "Message out of range", "Invalid (null) method", "Unknown message", "Manager call not supported", "Bad address", "Network operation in progress", "Network operation timed out", "Connection is busy", "Network attribute not supported", "Network error", "Address in use", "System out of memory", "Connection aborted", "Connection refused", "Not connected", "Already connected", "Connection closed", "Initialization error (interapplication manager)", "Bad occurrence", "Wait on unbound occurrence handler", "Occurrence queue overflow", "Datalog type conflict", "Unused", "Unrecognized type (interapplication manager)", "Memory corrupt", "Failed to make temporary DLL", "Old CIN version", "Drag socket not found", "Failed to load drop-object", "Failed to register OLE object", "Failed to release OLE object", "Format specifier type mismatch", "Unknown format specifier", "Too few format specifiers", "Too many format specifiers", "Scan failed", "Newer CIN version", "Error converting to variant", "Runtime menu error", "Password tampered", "Variant attribute not found", "Incompatible variant data type", "Event data is not available", "Event Store is not present", "Occurrence is not found", "Event Queue is not created", "Event info is not available", "Refnum passed is NULL", "Error retrieving Class GUID", "Error retrieving CoClass GUID", "Error retrieving TypeLib GUID.", "Bad built application magic bytes.", "Specific driver is different from the specific driver associated with the Logical Name.", "There is no session opened to the class driver.", "Max Error", "MAX - Error with config objects", "MAX - Error loading configuration", "MAX - Group not supported"]
        # "Handle mistyped state name (developer tool)"
        n137 = Format Into String(format string="Software Exception: Unhandled State \"%s\"." ("message"), error in=w293, w291) -> (resulting string=w296:string, error out=w295:errorcluster)  [unwired: 1 in]
        n138 = call <vilib>:"Error Cluster From Error Code.vi"("show call chain? (False)"=TRUE, "error in (no error)"=w295, "error message (\"\")"=w296, "error code (0)"=w297) -> ("error out"=w292:errorcluster)  [unwired: 5 in]
      }
      frame "Timeout" {
        # "High-Speed Measurement Stream"
        n139 = call "HPS-17000-PowerModule_GetAttributes.vi"("reference in"=w314, "Error In"=w313) -> ("Data"=w311:T10, "DataRef"=w307:refnum<data-value>, "Error Out"=w312:errorcluster)  [unwired: 10 in, 1 out]
        n140 = Unbundle By Name(w311) -> ("reserved"=w309:bool, "connected"=w310:bool, "measurement stream"=w306:bool, "HPS17000 Refs"=w305:refnum<class "HPS-17000.lvclass">[], "Configuration.Measurement Array Size"=w304:i32, "measurement array"=w303:T16[])
        n141 = case shown="False" w310 {
          tunnel: w312 -> [w315 w324]
          tunnel: [w315 w319] -> w308
          tunnel: w305 -> [_ w325]
          tunnel: w309 -> [_ w318]
          tunnel: w307 -> [_ w328]
          tunnel: w306 -> [_ w316]
          tunnel: w304 -> [_ w323]
          tunnel: w303 -> [_ w322]
          frame False {
          }
          frame True {
            n142 = Compound Arithmetic op=AND(w318, w316) -> (w317:bool)
            n143 = case shown="True" w317 {
              tunnel: w324 -> [w357 w367]
              tunnel: [w356 w362] -> w320
              tunnel: [w354 w363] -> w327
              tunnel: [w353 w360] -> w321
              tunnel: [w352 w358] -> w326
              tunnel: w325 -> [w355 w366]
              frame False {
                # "Connected, No Measurement Stream Started"
                n144 = call "TCP Read.vi"("error in (no error)"=w357, "HPS17000 Refs in"=w355) -> ("error out"=w356:errorcluster, "last timestamp"=w352:i64, "measurement array"=w353:T16[], "HPS17000 Refs out"=w354:refnum<class "HPS-17000.lvclass">[])  [unwired: 6 in]
              }
              frame True {
                # "Connected, Reserved, and UDP Measurement Stream OK"
                n145 = call "UDP Read.vi"("error in (no error)"=w367, "HPS17000 Refs in"=w366) -> ("error out"=w365:errorcluster, "last timestamp"=w359:i64, "measurement array"=w361:T16[], "HPS17000 Refs out"=w364:refnum<class "HPS-17000.lvclass">[])  [unwired: 6 in]
                n146 = case shown="Error .." w365 {
                  selector: w365 -> [w369 w379]
                  tunnel: w364 -> [w371 w376]
                  tunnel: [w371 w375] -> w363
                  tunnel: [w369 w374] -> w362
                  tunnel: w361 -> [w370 _]
                  tunnel: [w370 w372] -> w360
                  tunnel: w359 -> [w368 _]
                  tunnel: [w368 w373] -> w358
                  frame No Error {
                    # "UDP Read successful; continue."
                  }
                  frame Error {
                    # "-319827\nTimed out while\nreading stream"
                    # "Error reading UDP measurement stream; fallback to TCP read for this iteration."
                    n147 = call <vilib>:"Clear Errors.vi"("error in (no error)"=w379, "specific error code to clear (0: all)"=-319827 ("error code (0)")) -> ("error out"=w377:errorcluster)  [unwired: 4 in, 1 out]
                    n148 = call "TCP Read.vi"("error in (no error)"=w377, "HPS17000 Refs in"=w376) -> ("error out"=w374:errorcluster, "last timestamp"=w373:i64, "measurement array"=w372:T16[], "HPS17000 Refs out"=w375:refnum<class "HPS-17000.lvclass">[])  [unwired: 6 in]
                  }
                }
              }
            }
            n149 = case shown="No Error" w320 {
              selector: w320 -> [_ w351]
              tunnel: w328 -> [w336 _]
              tunnel: w327 -> [w335 _]
              tunnel: [w334 w351] -> w319
              tunnel: w326 -> [w333 _]
              tunnel: w323 -> [w332 _]
              tunnel: w322 -> [w331 _]
              tunnel: w321 -> [w329 _]
              frame No Error {
                n150 = in-place {
                  in-place-border: w332 -> [w340]
                  in-place-border: w329 -> [w337]
                  n151 = in-place-match #3(w331) -> (w339:T16[])
                  n152 = Insert Into Array(array=w339, new element=w337) -> (w343:T16[])  [unwired: 1 in]
                  n153 = Array Size(array=w343) -> (size(s)=w341:i32)
                  n154 = Subtract(x=w341, y=w340) -> (x-y=w344:i32)
                  n155 = Greater Than 0?(x=w344) -> (x > 0?=w342:bool)
                  n156 = Array Subset(array=w343, index=w344) -> (w345:T16[])  [unwired: 1 in]
                  n157 = Select(t=w345, s=w342, f=w343) -> (s? t:f=w338:T16[])
                  n158 = in-place-match #3(w338) -> (w330:T16[])
                }
                n159 = in-place {
                  in-place-border: w335 -> [w346]
                  in-place-border: w333 -> [w348]
                  in-place-border: w330 -> [w347]
                  n160 = in-place-dvr #4(w336) -> (w349:T10)  [unwired: 1 out]
                  n161 = Bundle By Name(cluster=w349, "HPS17000 Refs"=w346, "last timestamp"=w348, "measurement array"=w347) -> (w350:T10)
                  n162 = in-place-dvr #4(w350) -> (w334:errorcluster)  [unwired: 1 out]
                }
              }
              frame Error {
              }
            }
          }
        }
      }
      frame "Error Handler" {
        n163 = Unbundle By Name(w382) -> ("source"=w380:string)
        n164 = call <vilib>:"Write to System Log.vi"("message"=w380) -> ()  [unwired: 10 in, 1 out]
        "error info" <- w382
      }
      frame "Initialize Core Data" {
        # "Do not delete\nUsed by OpenGDS framework"
        # "Don't remove this property node\nit's necessary to keep front panel\nin memory for a built application."
        # "Template created by VI Technologies"
        n165 = local read "HPS17K IP Addresses"() -> (w386:string[])
        n166 = call "HPS-17000-PowerModule_GetAttributes.vi"("reference in"=w402, "Error In"=w399) -> ("reference out"=w400:refnum<class "HPS-17000-PowerModule.lvclass">, "Data"=w398:T10, "Error Out"=w401:errorcluster)  [unwired: 10 in, 1 out]
        n167 = Unbundle By Name(w398) -> ("Configuration.HPS17000 IP Addresses"=w387:string[], "Configuration.TSN NIC IP Address"=w397:string, "Configuration.HPS Topology"=w396:enum16{"SINGLE", "MULTI"}, "Configuration.Read Timeout (ms)"=w388:i32)
        n168 = for {
          tunnel: w386 -> [w415] mode=indexing
          tunnel: [w414] -> w385
          n169 = invoke on="HPS17K IP Addresses" class="Tree (strict)" method="Edit Tree Items.Delete"("tag"=w415) -> (error out=w414:errorcluster)  [unwired: 4 in, 4 out]
        }
        n170 = property on="reference in" class="LVClassControl (strict)" props=["Label", "Text"]() -> ()  [unwired: 2 in, 3 out]
        n171 = for {
          tunnel: w387 -> [w417] mode=indexing
          tunnel: w385 -> [w416]
          n172 = invoke on="HPS17K IP Addresses" class="Tree (strict)" method="Edit Tree Items.Add Item"(error in=w416, "Left Cell"=w417, "Child Tag"=w417) -> ()  [unwired: 6 in, 9 out]
        }
        n173 = local write "TSN NIC IP Address"(w397) -> ()
        n174 = local write "HPS Topology"(w396) -> ()
        n175 = call "ProcessRepository.vi"("reference in"=w400, "Error In"=w401) -> ("QueueFromProcess"=w405:refnum<queue>, "ProcessSyncQueue"=w403:refnum<queue>, "EventFromProcess"=w406:refnum<user-event>, "EventsToProcess"=w408:refnum<user-event>, "Error Out"=w409:errorcluster)  [unwired: 10 in, 3 out]
        n176 = register-events(error in=w409, w408) -> (reference out=w407:refnum<event-registration>, error out=w391:errorcluster)  [unwired: 1 in]
        n177 = Create User Event(user event datatype=string[][] [] ("HPS17000 Search Results"), error in=w391) -> (user event=w389:refnum<user-event>, error out=w390:errorcluster)
        n178 = Create User Event(user event datatype=FALSE ("Script Complete"), error in=w390) -> (user event=w394:refnum<user-event>, error out=w393:errorcluster)
        n179 = Enqueue Element(queue=w403, element="Started", error in (no error)=w393) -> (error out=w413:errorcluster)  [unwired: 1 in, 2 out]
        n180 = Bundle By Name(cluster=w410, "Core.Timeout"=w388, "Network Search Completed"=w389, "Self Test Completed"=w394, "Core.Events.EventsToProcess"=w407, "Core.EventFromProcess"=w406, "Core.ProcessSyncQueue"=w403, "Core.QueueFromProcess"=w405) -> (w411:T3)
      }
      frame "Data: Cleanup" {
        n181 = Unbundle By Name(w426) -> ("Core.ProcessSyncQueue"=w427:refnum<queue>, "Self Test Completed"=w420:refnum<user-event>, "Network Search Completed"=w422:refnum<user-event>, "Core.Events"=w424:T9)
        n182 = Unregister For Events(event registration refnum=w424, error in=w418) -> (error out=w423:errorcluster)
        n183 = Destroy User Event(user event=w422, error in=w423) -> (error out=w421:errorcluster)
        n184 = Destroy User Event(user event=w420, error in=w421) -> (error out=w419:errorcluster)
        n185 = flat-sequence {
          tunnel: [w433] -> w425
          tunnel: w427 -> [w432]
          tunnel: w419 -> [w431]
          frame #0 {
            n186 = Enqueue Element(queue=w432, element="Finished") -> (error out=w434:errorcluster)  [unwired: 2 in, 2 out]
            n187 = Merge Errors(w434, w431) -> (w433:errorcluster)
          }
        }
      }
      frame "Data: Update Periodic" {
        n188 = call "HPS-17000-PowerModule_GetAttributes.vi"("reference in"=w443, "Error In"=w442) -> ("Data"=w441:T10, "Error Out"=w439:errorcluster)  [unwired: 10 in, 2 out]
        n189 = Unbundle By Name(w441) -> ("measurement stream"=w435:bool, "setpoint stream"=w436:bool, "HPS17000 Refs"=w440:refnum<class "HPS-17000.lvclass">[], "connected"=w437:bool)
        n190 = case shown="True" w437 {
          tunnel: w440 -> [_ w449]
          tunnel: w439 -> [w446 w448]
          tunnel: [w446 w447] -> w438
          frame False {
          }
          frame True {
            n191 = call-poly <instrlib>:"Get Status.vi"("error in"=w448, "cycler refs in"=w449) -> ("error out"=w447:errorcluster, "heartbeat valid"=w451:bool[], "ok"=w452:bool)  [unwired: 6 in, 1 out]
            n192 = Index Array(array=w451) -> (element=w450:bool)  [unwired: 1 in]
            n193 = local write "Heartbeat Valid"(w450) -> ()
            n194 = local write "OK"(w452) -> ()
          }
        }
        n195 = local write "Measurement Stream"(w435) -> ()
        n196 = local write "Setpoint Stream"(w436) -> ()
      }
      frame "---------- UI ----------" {
      }
      frame "UI: Front Panel State" {
        n197 = case shown="\"Close\"" w457 {
          frame "Open", Default {
            n198 = property class="VI"() -> ("FP.State"=w460:T5)  [unwired: 2 in, 2 out]
            n199 = case shown="Default" w460 {
              frame Default {
                n200 = invoke class="VI" method="FP.Open"("Activate"=TRUE, "State"=T5."Standard") -> ()  [unwired: 3 in, 5 out]
              }
              frame "Standard" {
              }
            }
          }
          frame "Close" {
            n201 = property class="VI"() -> ("FP.State"=w463:T5)  [unwired: 2 in, 2 out]
            n202 = case shown="Default" w463 {
              frame "Closed" {
              }
              frame Default {
                n203 = invoke class="VI" method="FP.Close"() -> ()  [unwired: 3 in, 3 out]
              }
            }
          }
        }
      }
      frame "UI: Initialize" {
        w465 = string[][] [] ("Item Names")
        w468 = "" ("Device Search")
        w464 = string[] [] ("HPS17K IP Addresses")
        w469 = T6."Disabled and Grayed Out" ("Disabled")
        n204 = local write "HPS17K IP Addresses"(w464) -> ()
        n205 = local write "device properties"(T2 {"name"="", "model"="", "vendor"="", "serial_number"=""} ("device properties")) -> ()
        n206 = property on="Event Log" class="MCListbox (strict)"("ItemNames"=w465) -> ()  [unwired: 2 in, 2 out]
        n207 = property on="Hardware Limits" class="MCListbox (strict)"("ItemNames"=w465) -> ()  [unwired: 2 in, 2 out]
        n208 = property on="Temperatures" class="MCListbox (strict)"("ItemNames"=w465) -> ()  [unwired: 2 in, 2 out]
        n209 = property on="Thermal Limits" class="MCListbox (strict)"("ItemNames"=w465) -> ()  [unwired: 2 in, 2 out]
        n210 = property on="Test Server Log" class="LstBox (strict)"("Item Names"=w464) -> ()  [unwired: 2 in, 2 out]
        n211 = property on="Self Test Log" class="LstBox (strict)"("Item Names"=w464) -> ()  [unwired: 2 in, 2 out]
        n212 = property class="VI"() -> ("Name"=w484:string)  [unwired: 2 in, 2 out]
        n213 = local write "Main Tab Control"(T1."CONFIG" ("Main Tab Control")) -> ()
        n214 = Match Pattern(string=w484, regular expression="\\2Evi$") -> (before substring=w482:string)  [unwired: 1 in, 3 out]
        n215 = Reverse String(1:w482) -> (0:w481:string)
        n216 = Match Pattern(string=w481, regular expression=":") -> (before substring=w479:string, after substring=w477:string)  [unwired: 1 in, 2 out]
        n217 = Match Pattern(string=w477, regular expression="\\2E") -> (after substring=w475:string)  [unwired: 1 in, 3 out]
        n218 = property on="Get XC Report" class="Bool"("DisabledEnum"=w469) -> ()  [unwired: 2 in, 2 out]
        n219 = property on="FC Sys Inspect" class="Bool"("DisabledEnum"=w469) -> ()  [unwired: 2 in, 2 out]
        n220 = property on="Run Test Server" class="Bool (strict)"("DisabledEnum"=w469) -> ()  [unwired: 2 in, 2 out]
        n221 = property on="Run Self Test" class="Bool (strict)"("DisabledEnum"=w469) -> ()  [unwired: 2 in, 2 out]
        n222 = property on="Volta Monitor" class="Bool"("DisabledEnum"=w469) -> ()  [unwired: 2 in, 2 out]
        n223 = property on="Update Temperatures" class="Bool"("DisabledEnum"=w469) -> ()  [unwired: 2 in, 2 out]
        n224 = property on="Get Device Properties" class="Bool"("DisabledEnum"=w469) -> ()  [unwired: 2 in, 2 out]
        n225 = Reverse String(1:w479) -> (0:w473:string)
        n226 = Reverse String(1:w475) -> (0:w474:string)
        n227 = Format Into String(format string="%s %s", w474, w473) -> (resulting string=w472:string)  [unwired: 2 in, 1 out]
        n228 = local write "Voltage Reformation"(FALSE ("Voltage Reformation")) -> ()
        n229 = local write "Device Search"(w468) -> ()
        n230 = local write "GM ID"(w468) -> ()
        n231 = local write "Fault Description"(w468) -> ()
        n232 = property class="VI"("Front Panel.Title"=w472) -> ()  [unwired: 2 in, 2 out]
      }
      frame "UI: Cleanup" {
        n233 = property class="VI"() -> (error out=w487:errorcluster, "FP.State"=w489:T5)  [unwired: 2 in, 1 out]
        n234 = case shown="\"Standard\", Default" w489 {
          frame "Closed" {
          }
          frame "Standard", Default {
            n235 = invoke class="VI" method="FP.Close"() -> ()  [unwired: 3 in, 3 out]
          }
        }
      }
      frame "UI: Cursor Set" {
        # "Argument"
        # "Set and Unset Cursor Busy.\n(Usage: \"UI: Cursor Set >> Busy|Idle\")"
        n236 = disable-structure shown="TARGET_TYPE==Windows, Default" {
          disable-tunnel: w493 -> [w498 _]
          disable-tunnel: w492 -> [w497 w503]
          disable-tunnel: [w496 w503] -> w491
          frame condition #0 (active) {
            n237 = case shown="\"Busy\"" w498 {
              tunnel: w497 -> [w500 w502]
              tunnel: [w499 w501] -> w496
              frame "Idle", Default {
                n238 = call <vilib>:"Unset Busy.vi"("error in (no error)"=w500) -> ("error out"=w499:errorcluster)  [unwired: 10 in]
              }
              frame "Busy" {
                n239 = call <vilib>:"Set Busy.vi"("error in (no error)"=w502) -> ("error out"=w501:errorcluster)  [unwired: 9 in, 1 out]
              }
            }
          }
          frame condition #1 {
          }
        }
      }
      frame "---------- CMD ----------" {
      }
      frame "CMD: Connect" {
        w507 = T6."Enabled" ("Disabled")
        n240 = property on="Get XC Report" class="Bool"("DisabledEnum"=w507) -> ()  [unwired: 2 in, 2 out]
        n241 = property on="FC Sys Inspect" class="Bool"("DisabledEnum"=w507) -> ()  [unwired: 2 in, 2 out]
        n242 = property on="Run Test Server" class="Bool (strict)"("DisabledEnum"=w507) -> ()  [unwired: 2 in, 2 out]
        n243 = property on="Volta Monitor" class="Bool"("DisabledEnum"=w507) -> ()  [unwired: 2 in, 2 out]
        n244 = property on="Update Temperatures" class="Bool"("DisabledEnum"=w507) -> ()  [unwired: 2 in, 2 out]
        n245 = property on="Get Device Properties" class="Bool"("DisabledEnum"=w507) -> ()  [unwired: 2 in, 2 out]
      }
      frame "CMD: Disconnect" {
        w511 = T6."Disabled and Grayed Out" ("Disabled")
        n246 = property on="Get XC Report" class="Bool"("DisabledEnum"=w511) -> ()  [unwired: 2 in, 2 out]
        n247 = property on="FC Sys Inspect" class="Bool"("DisabledEnum"=w511) -> ()  [unwired: 2 in, 2 out]
        n248 = property on="Run Test Server" class="Bool (strict)"("DisabledEnum"=w511) -> ()  [unwired: 2 in, 2 out]
        n249 = property on="Volta Monitor" class="Bool"("DisabledEnum"=w511) -> ()  [unwired: 2 in, 2 out]
        n250 = property on="Update Temperatures" class="Bool"("DisabledEnum"=w511) -> ()  [unwired: 2 in, 2 out]
        n251 = property on="Get Device Properties" class="Bool"("DisabledEnum"=w511) -> ()  [unwired: 2 in, 2 out]
        n252 = property on="Run Self Test" class="Bool (strict)"("DisabledEnum"=w511) -> ()  [unwired: 2 in, 2 out]
      }
      frame "CMD: Reserve" {
        # "Reserve Macro\n(This is called when we reserve the HPS17K)"
        n253 = call <vilib>:"Add State(s) to Queue__jki_lib_state_machine.vi"("State(s) in Front (\"\")"="CMD: Start Measurement Stream\nCMD: Read Thermal Limits\nCMD: Read Hardware Limits\nCMD: Read Temperatures", "State(s) in (\"\")"=w517) -> ("States Out"=w516:string)  [unwired: 13 in]
      }
      frame "CMD: Unreserve" {
        # "Unreserve Macro\n(This is called when we unreserve the HPS17K)"
        n254 = call <vilib>:"Add State(s) to Queue__jki_lib_state_machine.vi"("State(s) in Front (\"\")"="CMD: Stop Measurement Stream", "State(s) in (\"\")"=w522) -> ("States Out"=w521:string)  [unwired: 13 in]
      }
      frame "CMD: Exit" {
      }
      frame "CMD: Front Panel State" {
        n255 = Format Into String(format string="UI: Front Panel State>>%s" ("string"), w529) -> (resulting string=w528:string)  [unwired: 2 in, 1 out]
        n256 = call <vilib>:"Add State(s) to Queue__jki_lib_state_machine.vi"("State(s) in (\"\")"=w532, "State(s) at Back (\"\")"=w528) -> ("States Out"=w531:string)  [unwired: 13 in]
      }
      frame "CMD: Register Events" {
        n257 = call "HPS-17000-PowerModule_GetAttributes.vi"("reference in"=w540, "Error In"=w539) -> ("Data"=w537:T10, "Error Out"=w538:errorcluster)  [unwired: 10 in, 2 out]
        n258 = Unbundle By Name(w545) -> ("Self Test Completed"=w543:refnum<user-event>, "Network Search Completed"=w542:refnum<user-event>)
        n259 = Unbundle By Name(w537) -> ("GM ID"=w536:string, "events"=w535:T13)
        n260 = register-events(error in=w538, w535, w543, w542) -> (reference out=w541:refnum<event-registration>, error out=w546:errorcluster)  [unwired: 1 in]
        n261 = local write "GM ID"(w536) -> ()
        n262 = Bundle By Name(cluster=w545, "Core.Events.UserEvents"=w541) -> (w544:T3)
      }
      frame "CMD: Start Test Server" {
        n263 = Unbundle By Name(w549) -> ("Test Server"=w550:refnum<class "SSH.lvclass">)
        n264 = Equal?(x=refnum<class "SSH.lvclass"> refnum, y=w550) -> (x = y?=w551:bool)
        n265 = case shown="True" w551 {
          tunnel: w554 -> [w557 w568]
          tunnel: [w557 w569] -> w553
          tunnel: w550 -> [_ _]
          tunnel: w549 -> [w556 w563]
          tunnel: [w556 w562] -> w548
          frame False {
          }
          frame True {
            w565 = "~/testserver.log" ("format string")
            w566 = 1000  # Update Rate (ms)
            n266 = property on="HPS17K IP Addresses" class="Tree (strict)"() -> ("All Tags"=w558:string[])  [unwired: 2 in, 2 out]
            n267 = Index Array(array=w558) -> (element=w560:string)  [unwired: 1 in]
            n268 = control-ref of="Test Server Log"() -> (w559:refnum<vi>)
            n269 = property on="Run Self Test" class="Bool (strict)"("DisabledEnum"=T6."Enabled" ("Disabled")) -> ()  [unwired: 2 in, 2 out]
            n270 = Format Into String(format string="script -c ~/testserver.sh -f %s", w565) -> (resulting string=w567:string)  [unwired: 2 in, 1 out]
            n271 = call "SSH_Create.vi"("Full Command"=w567, "Script Name"="pess_testsuite_" ("format string"), "Log File"=w565, "IP Address"=w560, "Error In"=w568, "Update Rate (ms)"=w566, "Console Listbox"=w559) -> ("reference out"=w561:refnum<class "SSH.lvclass">, "Error Out"=w569:errorcluster)  [unwired: 11 in]
            n272 = Bundle By Name(cluster=w563, "Test Server"=w561) -> (w562:T3)
          }
        }
      }
      frame "CMD: Start Self Test" {
        n273 = Unbundle By Name(w578) -> ("Self Test"=w574:refnum<class "SSH.lvclass">, "Self Test Completed"=w573:refnum<user-event>)
        n274 = Equal?(x=refnum<class "SSH.lvclass"> refnum, y=w574) -> (x = y?=w575:bool)
        n275 = case shown="True" w575 {
          tunnel: w581 -> [w584 w585]
          tunnel: [w584 w598] -> w580
          tunnel: [w583 w599] -> w576
          tunnel: w574 -> [w583 _]
          tunnel: w573 -> [_ w586]
          tunnel: "Voltage Reformation" -> [_ w593]
          frame False {
          }
          frame True {
            w594 = "~/selftest.log" ("format string")
            n276 = Select(t="~/selftest-reform.sh" ("format string"), s=w593, f="~/selftest.sh" ("format string")) -> (s? t:f=w591:string)
            n277 = property on="HPS17K IP Addresses" class="Tree (strict)"() -> ("All Tags"=w587:string[])  [unwired: 2 in, 2 out]
            n278 = Format Into String(format string="script -c %s -f %s", w591, w594) -> (resulting string=w596:string)  [unwired: 2 in, 1 out]
            n279 = control-ref of="Self Test Log"() -> (w589:refnum<vi>)
            n280 = Index Array(array=w587) -> (element=w588:string)  [unwired: 1 in]
            n281 = call "SSH_Create.vi"("Full Command"=w596, "Script Name"="pess_selftest" ("format string"), "Log File"=w594, "IP Address"=w588, "Error In"=w585, "Update Rate (ms)"=1000, "Console Listbox"=w589, "Script Complete Event"=w586) -> ("reference out"=w599:refnum<class "SSH.lvclass">, "Error Out"=w598:errorcluster)  [unwired: 10 in]
          }
        }
        n282 = Bundle By Name(cluster=w578, "Self Test"=w576) -> (w579:T3)
      }
      frame "CMD: Start Measurement Stream" {
        n283 = call "HPS-17000-PowerModule_GetAttributes.vi"("reference in"=w605, "Error In"=w604) -> ("DataRef"=w603:refnum<data-value>, "Error Out"=w602:errorcluster)  [unwired: 10 in, 2 out]
        n284 = in-place {
          in-place-border: w602 -> [w618]
          in-place-border: [w611] -> w601
          n285 = in-place-dvr #5(w603) -> (w617:T10)  [unwired: 1 out]
          n286 = Unbundle By Name(w617) -> ("connected"=w609:bool, "reserved"=w610:bool, "HPS17000 Refs"=w616:refnum<class "HPS-17000.lvclass">[], "last timestamp"=w613:i64)
          n287 = Add(x=w613, y=i64 1000000000) -> (x+y=w612:i64)
          n288 = And(x=w609, y=w610) -> (x .and. y?=w608:bool)
          n289 = To Unsigned Quad Integer(1:w612) -> (0:w614:u64)
          n290 = case shown="True" w608 {
            tunnel: [w621 w630] -> w619
            tunnel: w618 -> [w620 w629]
            tunnel: w617 -> [w621 w628]
            tunnel: w616 -> [_ w626]
            tunnel: w614 -> [_ w625]
            tunnel: [w620 w622] -> w611
            frame False {
            }
            frame True {
              n291 = call-poly <instrlib>:"Start Measurement Stream.vi"("error in"=w629, "start timestamp"=w625, "cycler refs in"=w626) -> ("error out"=w622:errorcluster, "cycler refs out"=w627:refnum<class "HPS-17000.lvclass">[])  [unwired: 7 in]
              n292 = Unbundle By Name(w622) -> ("status"=w624:bool)
              n293 = Not(x=w624) -> (.not. x?=w623:bool)
              n294 = Bundle By Name(cluster=w628, "HPS17000 Refs"=w627, "measurement stream"=w623) -> (w630:T10)
            }
          }
          n295 = in-place-dvr #5(w619) -> ()  [unwired: 2 out]
        }
      }
      frame "CMD: Start Setpoint Stream" {
        n296 = call "HPS-17000-PowerModule_GetAttributes.vi"("reference in"=w635, "Error In"=w634) -> ("DataRef"=w633:refnum<data-value>, "Error Out"=w632:errorcluster)  [unwired: 10 in, 2 out]
        n297 = in-place {
          in-place-border: w632 -> [w645]
          in-place-border: [w642] -> w631
          n298 = in-place-dvr #6(w633) -> (w644:T10)  [unwired: 1 out]
          n299 = Unbundle By Name(w644) -> ("connected"=w640:bool, "reserved"=w639:bool, "HPS17000 Refs"=w643:refnum<class "HPS-17000.lvclass">[], "Configuration.Setpoint Stream Config"=w641:T12)
          n300 = And(x=w640, y=w639) -> (x .and. y?=w638:bool)
          n301 = case shown="True" w638 {
            tunnel: [w648 w657] -> w646
            tunnel: w645 -> [w647 w656]
            tunnel: w644 -> [w648 w655]
            tunnel: w643 -> [_ w653]
            tunnel: [w647 w652] -> w642
            tunnel: w641 -> [_ w651]
            frame False {
            }
            frame True {
              n302 = call-poly <instrlib>:"Start Setpoint Stream.vi"("error in"=w656, "setpoint stream config"=w651, "cycler refs in"=w653) -> ("error out"=w652:errorcluster, "cycler refs out"=w654:refnum<class "HPS-17000.lvclass">[])  [unwired: 7 in]
              n303 = Unbundle By Name(w652) -> ("status"=w650:bool)
              n304 = Not(x=w650) -> (.not. x?=w649:bool)
              n305 = Bundle By Name(cluster=w655, "HPS17000 Refs"=w654, "setpoint stream"=w649) -> (w657:T10)
            }
          }
          n306 = in-place-dvr #6(w646) -> ()  [unwired: 2 out]
        }
      }
      frame "CMD: Update Setpoint Stream" {
        n307 = call "HPS-17000-PowerModule_GetAttributes.vi"("reference in"=w662, "Error In"=w661) -> ("DataRef"=w660:refnum<data-value>, "Error Out"=w659:errorcluster)  [unwired: 10 in, 2 out]
        n308 = in-place {
          in-place-border: w659 -> [w672]
          in-place-border: [w668] -> w658
          # "#TODO UPDATE THIS WITH CORRECT SETPOINTS AND dT"
          n309 = in-place-dvr #7(w660) -> (w671:T10)  [unwired: 1 out]
          n310 = Unbundle By Name(w671) -> ("last timestamp"=w667:i64, "HPS17000 Refs"=w669:refnum<class "HPS-17000.lvclass">[])
          n311 = call-poly <instrlib>:"Stream Setpoints.vi"("dt"=i64 0, "t0"=w667, "error in"=w672, "setpoints"=T7[] [], "cycler refs in"=w669) -> ("error out"=w668:errorcluster, "cycler refs out"=w670:refnum<class "HPS-17000.lvclass">[])  [unwired: 5 in]
          n312 = Bundle By Name(cluster=w671, "HPS17000 Refs"=w670) -> (w673:T10)
          n313 = in-place-dvr #7(w673) -> ()  [unwired: 2 out]
        }
      }
      frame "CMD: Stop Setpoint Stream" {
        n314 = call "HPS-17000-PowerModule_GetAttributes.vi"("reference in"=w678, "Error In"=w677) -> ("DataRef"=w676:refnum<data-value>, "Error Out"=w675:errorcluster)  [unwired: 10 in, 2 out]
        n315 = in-place {
          in-place-border: w675 -> [w687]
          in-place-border: [w684] -> w674
          n316 = in-place-dvr #8(w676) -> (w686:T10)  [unwired: 1 out]
          n317 = Unbundle By Name(w686) -> ("connected"=w682:bool, "reserved"=w683:bool, "HPS17000 Refs"=w685:refnum<class "HPS-17000.lvclass">[])
          n318 = And(x=w682, y=w683) -> (x .and. y?=w681:bool)
          n319 = case shown="True" w681 {
            tunnel: [w690 w697] -> w688
            tunnel: w687 -> [w689 w696]
            tunnel: w686 -> [w690 w695]
            tunnel: w685 -> [_ w693]
            tunnel: [w689 w692] -> w684
            frame False {
            }
            frame True {
              n320 = call-poly <instrlib>:"Stop Setpoint Stream.vi"("error in"=w696, "cycler refs in"=w693) -> ("error out"=w692:errorcluster, "cycler refs out"=w694:refnum<class "HPS-17000.lvclass">[])  [unwired: 8 in]
              n321 = Unbundle By Name(w692) -> ("status"=w691:bool)
              n322 = Bundle By Name(cluster=w695, "HPS17000 Refs"=w694, "setpoint stream"=w691) -> (w697:T10)
            }
          }
          n323 = in-place-dvr #8(w688) -> ()  [unwired: 2 out]
        }
      }
      frame "CMD: Stop Measurement Stream" {
        n324 = call "HPS-17000-PowerModule_GetAttributes.vi"("reference in"=w702, "Error In"=w701) -> ("DataRef"=w700:refnum<data-value>, "Error Out"=w699:errorcluster)  [unwired: 10 in, 2 out]
        n325 = in-place {
          in-place-border: w699 -> [w711]
          in-place-border: [w709] -> w698
          n326 = in-place-dvr #9(w700) -> (w713:T10)  [unwired: 1 out]
          n327 = Unbundle By Name(w713) -> ("HPS17000 Refs"=w712:refnum<class "HPS-17000.lvclass">[], "connected"=w706:bool, "reserved"=w705:bool)
          n328 = And(x=w706, y=w705) -> (x .and. y?=w707:bool)
          n329 = case shown="True" w707 {
            tunnel: w712 -> [w717 w722]
            tunnel: w711 -> [w716 w721]
            tunnel: [w717 w720] -> w710
            tunnel: [w716 w719] -> w709
            tunnel: [FALSE ("status") w718] -> w708
            frame False {
            }
            frame True {
              n330 = call-poly <instrlib>:"Stop Measurement Stream.vi"("error in"=w721, "cycler refs in"=w722) -> ("error out"=w719:errorcluster, "cycler refs out"=w720:refnum<class "HPS-17000.lvclass">[])  [unwired: 8 in]
              n331 = Unbundle By Name(w719) -> ("status"=w718:bool)
            }
          }
          n332 = Bundle By Name(cluster=w713, "HPS17000 Refs"=w710, "measurement stream"=w708) -> (w714:T10)
          n333 = in-place-dvr #9(w714) -> ()  [unwired: 2 out]
        }
      }
      frame "CMD: Stop Self Test" {
        n334 = Unbundle By Name(w723) -> ("Self Test"=w726:refnum<class "SSH.lvclass">)
        n335 = Equal?(x=refnum<class "SSH.lvclass"> refnum, y=w726) -> (x = y?=w728:bool)
        n336 = case shown="False" w728 {
          tunnel: w729 -> [w736 w737]
          tunnel: w726 -> [w735 _]
          tunnel: [w734 w737] -> w725
          tunnel: w723 -> [w733 w738]
          tunnel: [w732 w738] -> w724
          frame False {
            n337 = call-dynamic "Destroy.vi"("reference in"=w735, "Error In"=w736) -> ("Error Out"=w734:errorcluster)  [unwired: 16 in, 1 out]
            n338 = Bundle By Name(cluster=w733, "Self Test"=refnum<class "SSH.lvclass"> refnum) -> (w732:T3)
          }
          frame True {
          }
        }
      }
      frame "CMD: Stop Test Server" {
        n339 = Unbundle By Name(w739) -> ("Test Server"=w742:refnum<class "SSH.lvclass">)
        n340 = Equal?(x=refnum<class "SSH.lvclass"> refnum, y=w742) -> (x = y?=w744:bool)
        n341 = case shown="False" w744 {
          tunnel: w745 -> [w753 w754]
          tunnel: w742 -> [w752 _]
          tunnel: [w751 w754] -> w741
          tunnel: w739 -> [w750 w755]
          tunnel: [w749 w755] -> w740
          frame False {
            n342 = call-dynamic "Destroy.vi"("reference in"=w752, "Error In"=w753) -> ("Error Out"=w751:errorcluster)  [unwired: 16 in, 1 out]
            n343 = property on="Run Self Test" class="Bool (strict)"("DisabledEnum"=T6."Disabled and Grayed Out" ("Disabled")) -> ()  [unwired: 2 in, 2 out]
            n344 = Bundle By Name(cluster=w750, "Test Server"=refnum<class "SSH.lvclass"> refnum ("Self Test")) -> (w749:T3)
          }
          frame True {
          }
        }
      }
      frame "CMD: Read Thermal Limits" {
        n345 = property on="HPS17K IP Addresses" class="Tree (strict)"() -> ("All Tags"=w756:string[])  [unwired: 2 in, 2 out]
        n346 = Index Array(array=w756) -> (element=w759:string)  [unwired: 1 in]
        n347 = call "Get MB Registers.vi"("error in (no error)"=w758, "Register Names"=string[] ["LIM_TEMP_AIR", "LIM_TEMP_TR", "T_AIR_LOW", "T_AIR_HIGH", "T_TR_LOW", "T_TR_HIGH"], "HPS17K IP Address"=w759) -> ("error out"=w757:errorcluster, "Register Data"=w761:string[][])  [unwired: 7 in]
        n348 = property on="Thermal Limits" class="MCListbox (strict)"("ItemNames"=w761) -> ()  [unwired: 2 in, 2 out]
      }
      frame "CMD: Read Hardware Limits" {
        n349 = property on="HPS17K IP Addresses" class="Tree (strict)"() -> ("All Tags"=w764:string[])  [unwired: 2 in, 2 out]
        n350 = Index Array(array=w764) -> (element=w768:string)  [unwired: 1 in]
        n351 = call "Get MB Registers.vi"("error in (no error)"=w766, "Register Names"=string[] ["LIM_HW_I_PARALLEL_POS", "LIM_HW_I_PARALLEL_NEG", "LIM_HW_I_SERIES_POS", "LIM_HW_I_SERIES_NEG", "LIM_HW_V_PARALLEL_HIGH", "LIM_HW_V_PARALLEL_LOW", "LIM_HW_V_SERIES_HIGH", "LIM_HW_V_SERIES_LOW", "LIM_HW_P_POS", "LIM_HW_P_NEG", "LIM_HW_R_HIGH", "LIM_HW_R_LOW"], "HPS17K IP Address"=w768) -> ("error out"=w765:errorcluster, "Register Data"=w769:string[][])  [unwired: 7 in]
        n352 = property on="Hardware Limits" class="MCListbox (strict)"("ItemNames"=w769) -> ()  [unwired: 2 in, 2 out]
      }
      frame "CMD: Read Temperatures" {
        n353 = property on="HPS17K IP Addresses" class="Tree (strict)"() -> ("All Tags"=w772:string[])  [unwired: 2 in, 2 out]
        n354 = Index Array(array=w772) -> (element=w773:string)  [unwired: 1 in]
        n355 = call "Get MB Registers.vi"("error in (no error)"=w777, "Register Names"=string[] ["bo_rear", "bo_front", "cc_rear", "cc_front", "trafo1/0", "trafo1/1", "trafo1/2", "trafo2/0", "trafo2/1", "trafo2/2"], "HPS17K IP Address"=w773) -> ("error out"=w776:errorcluster, "Register Data"=w775:string[][])  [unwired: 7 in]
        n356 = property on="Temperatures" class="MCListbox (strict)"("ItemNames"=w775) -> ()  [unwired: 2 in, 2 out]
      }
      frame "CMD: Write Slew Rates" {
        n357 = Unbundle By Name(w794) -> ("Core.QueueFromProcess"=w787:refnum<queue>, "Core.Data"=w793:variant)
        n358 = property on="HPS17K IP Addresses" class="Tree (strict)"() -> ("All Tags"=w780:string[])  [unwired: 2 in, 2 out]
        n359 = Variant To Data(error in=w795, type=T8 {"Current Decrease (A/sec)"=0.0, "Current Increase (A/sec)"=0.0, "Voltage Decrease (V/sec)"=0.0, "Voltage Increase (V/sec)"=0.0, "Resistance Decrease (Ohm/sec)"=0.0, "Resistance Increase (Ohm/sec)"=0.0} ("Slew Rates"), Variant=w793) -> (data=w790:T8, error out=w792:errorcluster)
        n360 = Index Array(array=w780) -> (element=w796:string)  [unwired: 1 in]
        n361 = Cluster To Array(cluster=w790) -> (array=w789:dbl[])
        n362 = call "Set MB Registers.vi"("error in (no error)"=w792, "Register Data"=w789, "Register Names"=string[] ["RATE_LIM_SP_V_INC", "RATE_LIM_SP_V_DEC", "RATE_LIM_SP_I_INC", "RATE_LIM_SP_I_DEC", "RATE_LIM_SP_R_INC", "RATE_LIM_SP_R_DEC"], "HPS17K IP Address"=w796) -> ("error out"=w784:errorcluster, "Register Data"=w786:string[][])  [unwired: 6 in]
        n363 = Array To Spreadsheet String(delimiter (Tab)=",", array=w786, 3:"%s" ("format string")) -> (spreadsheet string=w783:string)
        n364 = Enqueue Element(queue=w787, element=w783, error in (no error)=w784) -> (error out=w782:errorcluster)  [unwired: 1 in, 2 out]
      }
      frame "CMD: Read Slew Rates" {
        n365 = Unbundle By Name(w819) -> ("Core.QueueFromProcess"=w818:refnum<queue>)
        n366 = property on="HPS17K IP Addresses" class="Tree (strict)"() -> ("All Tags"=w798:string[])  [unwired: 2 in, 2 out]
        n367 = Index Array(array=w798) -> (element=w816:string)  [unwired: 1 in]
        n368 = call "Get MB Registers.vi"("error in (no error)"=w814, "Register Names"=string[] ["RATE_LIM_SP_V_INC", "RATE_LIM_SP_V_DEC", "RATE_LIM_SP_I_INC", "RATE_LIM_SP_I_DEC", "RATE_LIM_SP_R_INC", "RATE_LIM_SP_R_DEC"], "HPS17K IP Address"=w816) -> ("error out"=w812:errorcluster, "Register Data"=w808:string[][])  [unwired: 7 in]
        n369 = Index Array(array=w808, index (col)=1 ("disabled index (col)")) -> (element=w806:string[])  [unwired: 1 in]
        n370 = Fract/Exp String To Number(string=w806) -> (number=w805:dbl[])  [unwired: 3 in, 1 out]
        n371 = Index Array(array=w805) -> (element #1=w804:dbl, element #2=w803:dbl, element #3=w802:dbl, element #4=w801:dbl, element #5=w800:dbl, element #6=w799:dbl)  [unwired: 6 in]
        n372 = Bundle By Name(cluster=T8 {"Current Decrease (A/sec)"=0.0, "Current Increase (A/sec)"=0.0, "Voltage Decrease (V/sec)"=0.0, "Voltage Increase (V/sec)"=0.0, "Resistance Decrease (Ohm/sec)"=0.0, "Resistance Increase (Ohm/sec)"=0.0} ("Slew Rates"), "Voltage Increase (V/sec)"=w804, "Voltage Decrease (V/sec)"=w803, "Current Increase (A/sec)"=w802, "Current Decrease (A/sec)"=w801, "Resistance Increase (Ohm/sec)"=w800, "Resistance Decrease (Ohm/sec)"=w799) -> (w810:T8)
        n373 = Flatten To String(anything=w810, error in (no error)=w812) -> (data string=w809:string, error out=w811:errorcluster)  [unwired: 2 in, 1 out]
        n374 = Enqueue Element(queue=w818, element=w809, error in (no error)=w811) -> (error out=w817:errorcluster)  [unwired: 1 in, 2 out]
      }
      frame "CMD: Search HPS Network" {
        w832 = 128  # call and forget
        n375 = Unbundle By Name(w823) -> ("Network Search Completed"=w821:refnum<user-event>)
        n376 = vi-ref "HPS-17000-PowerModule.lvlib:HPS-17000-PowerModule.lvclass:Search HPS Network.vi"() -> (w834:refnum<vi>)
        n377 = property class="VI Interface Type 1"(reference=w834, error in=w822) -> (reference out=w830:refnum<vi>, error out=w833:errorcluster, "Path"=w831:path)
        n378 = local read "Controller TSN IP"() -> (w826:string)
        n379 = Open VI Reference(type specifier VI Refnum (for type only)=w830, vi path=w831, options=w832, error in (no error)=w833) -> (vi reference=w828:refnum<vi>, error out=w829:errorcluster)  [unwired: 2 in]
        n380 = call-by-ref "Start Asynchronous Call"(reference=w828, error in=w829, "reference in"=w827, "Controller TSN IP"=w826, "Network Search Completed"=w821) -> (error out=w825:errorcluster)  [unwired: 11 in, 3 out]
      }
      frame "CMD: Acknowledge" {
        n381 = local write "Fault Description"("" ("Fault Description")) -> ()
      }
      frame "---------- Macro ----------" {
      }
      frame "Macro: Initialize" {
        n382 = call <vilib>:"Add State(s) to Queue__jki_lib_state_machine.vi"("State(s) in Front (\"\")"="Initialize Core Data\nCMD: Register Events\nUI: Initialize" ("States Out"), "State(s) in (\"\")"=w844) -> ("States Out"=w842:string)  [unwired: 13 in]
      }
      frame "Macro: Start Test Server" {
        # "Start Test Server Macro\n(This is called when we start the test server on the HPS17K)"
        n383 = call <vilib>:"Add State(s) to Queue__jki_lib_state_machine.vi"("State(s) in Front (\"\")"="UI: Cursor Set >> Busy\nCMD: Start Test Server\nUI: Cursor Set >> Idle", "State(s) in (\"\")"=w849) -> ("States Out"=w848:string)  [unwired: 13 in]
      }
      frame "Macro: Search HPS Network" {
        # "Search HPS Network Macro\n(This is called when we search the network for HPS17K devices)"
        n384 = call <vilib>:"Add State(s) to Queue__jki_lib_state_machine.vi"("State(s) in Front (\"\")"="UI: Cursor Set >> Busy\nCMD: Search HPS Network\nUI: Cursor Set >> Idle", "State(s) in (\"\")"=w854) -> ("States Out"=w853:string)  [unwired: 13 in]
      }
      frame "Macro: Stop Test Server" {
        # "Stop Test Server Macro\n(This is called when we stop the test server on the HPS17K)"
        n385 = call <vilib>:"Add State(s) to Queue__jki_lib_state_machine.vi"("State(s) in Front (\"\")"="UI: Cursor Set >> Busy\nCMD: Stop Self Test\nCMD: Stop Test Server\nUI: Cursor Set >> Idle", "State(s) in (\"\")"=w859) -> ("States Out"=w858:string)  [unwired: 13 in]
      }
      frame "Macro: Start Self Test" {
        # "Start Self Test Macro\n(This is called when we start the self test on the HPS17K)"
        n386 = call <vilib>:"Add State(s) to Queue__jki_lib_state_machine.vi"("State(s) in Front (\"\")"="UI: Cursor Set >> Busy\nCMD: Start Self Test\nEvents: Register \nUI: Cursor Set >> Idle", "State(s) in (\"\")"=w864) -> ("States Out"=w863:string)  [unwired: 13 in]
      }
      frame "Macro: Stop Self Test" {
        # "Stop Self Test Macro\n(This is called when we start the self test on the HPS17K)"
        n387 = call <vilib>:"Add State(s) to Queue__jki_lib_state_machine.vi"("State(s) in Front (\"\")"="UI: Cursor Set >> Busy\nCMD: Stop Self Test\nUI: Cursor Set >> Idle", "State(s) in (\"\")"=w869) -> ("States Out"=w868:string)  [unwired: 13 in]
      }
      frame "Macro: Start Setpoint Stream" {
        # "Start Setpoint Stream Macro\n(This is called when we start the setpoint stream)"
        n388 = call <vilib>:"Add State(s) to Queue__jki_lib_state_machine.vi"("State(s) in Front (\"\")"="UI: Cursor Set >> Busy\nCMD: Start Setpoint Stream\nCMD: Update Setpoint Stream\nUI: Cursor Set >> Idle", "State(s) in (\"\")"=w874) -> ("States Out"=w873:string)  [unwired: 13 in]
      }
      frame "Macro: Stop Setpoint Stream" {
        # "Stop Setpoint Stream Macro\n(This is called when we stop the setpoint stream)"
        n389 = call <vilib>:"Add State(s) to Queue__jki_lib_state_machine.vi"("State(s) in Front (\"\")"="UI: Cursor Set >> Busy\nHPS: Stop Setpoint Stream\nUI: Cursor Set >> Idle", "State(s) in (\"\")"=w879) -> ("States Out"=w878:string)  [unwired: 13 in]
      }
      frame "Macro: Exit" {
        # "Exit Macro\n(This is called once, when the VI exits)"
        n390 = call <vilib>:"Add State(s) to Queue__jki_lib_state_machine.vi"("State(s) in Front (\"\")"="CMD: Stop Self Test\nCMD: Stop Test Server\nUI: Cleanup\nData: Cleanup" ("State(s) at Back (\"\")"), "State(s) in (\"\")"=w884) -> ("States Out"=w883:string)  [unwired: 13 in]
      }
    }
  }
  "error out" <- w5
  "reference out" <- "reference in"
